vi "Laser engraver main.vi"() -> ()   [LabVIEW 2016]
uses:
  Control panel.ctl
  Data.ctl
  <vilib>/LabVIEW Interface for Arduino/Type Defs/Arduino Resource.ctl
  <vilib>/LabVIEW Interface for Arduino/Type Defs/Board Type.ctl
  States.ctl
  <vilib>/Utility/file.llb/Write Delimited Spreadsheet (string).vi
  <vilib>/LabVIEW Interface for Arduino/LabVIEW Interface for Arduino.lvlib
panel:
  in  "Szimuláció ON/OFF 4":bool
  in  "Szimuláció ON/OFF 3":bool
  in  "Szimuláció ON/OFF 2":bool
  in  "Tab Control 2":T1(tab)
  in  "Kép elhelyezése":bool
  in  "Szimuláció ON/OFF":bool
  in  "Megmunkálás":bool
  in  "Program leállítása":bool
  in  "Kezelõpult":T2={"Konverziós faktor"=1020, "Threshold"=1020, "Megjegyzések"="", "Lépés"=0, "Sebesség"=0, " X init"=0, "Y init"=0} {"Y init" min=0; "X init" min=0; "Threshold" scale=0.0..16777215.0; "Konverziós faktor" scale=1.0..100.0}
  in  "Kilépés a programból":bool
  in  "VISA resource":refnum<visa-resource-name>
  in  "Képfeldolgozás":bool
  in  "Megmunkálás leállítása":bool
  in  "Felfüggesztés/Folytatás":bool
  out "Megmunkálás kész":bool
  out "Inicializálás a kezdõpontra":bool
  out "Megmunkálás folyamatban":bool
  in  "Tab Control":T3(tab)
  out "Eredeti kép":picture
  out "Fekete-fehér tükrözött kép":picture
  out "régi x felbontás":i16
  out "régi y felbontás":i16
  out "új x felbontás / oszlopok száma":i32
  out "új y felbontás / sorok száma":i32
  out "XY Graph 2":cluster{i32[], i32[]}[](graph)
  out "XY Graph":cluster{i32, i32}[](graph)
  in  "Kép beolvasása":bool
  in  "Kezelõpult betöltése":bool
  in  "Kezelõpult mentése":bool
  in  "Szélek kijelölése":bool
  in  "Jegyzõkönyvezés":bool
  # "Lézeres gravírozás\n\nLabview-ban implementálta:\nTari Balázs"
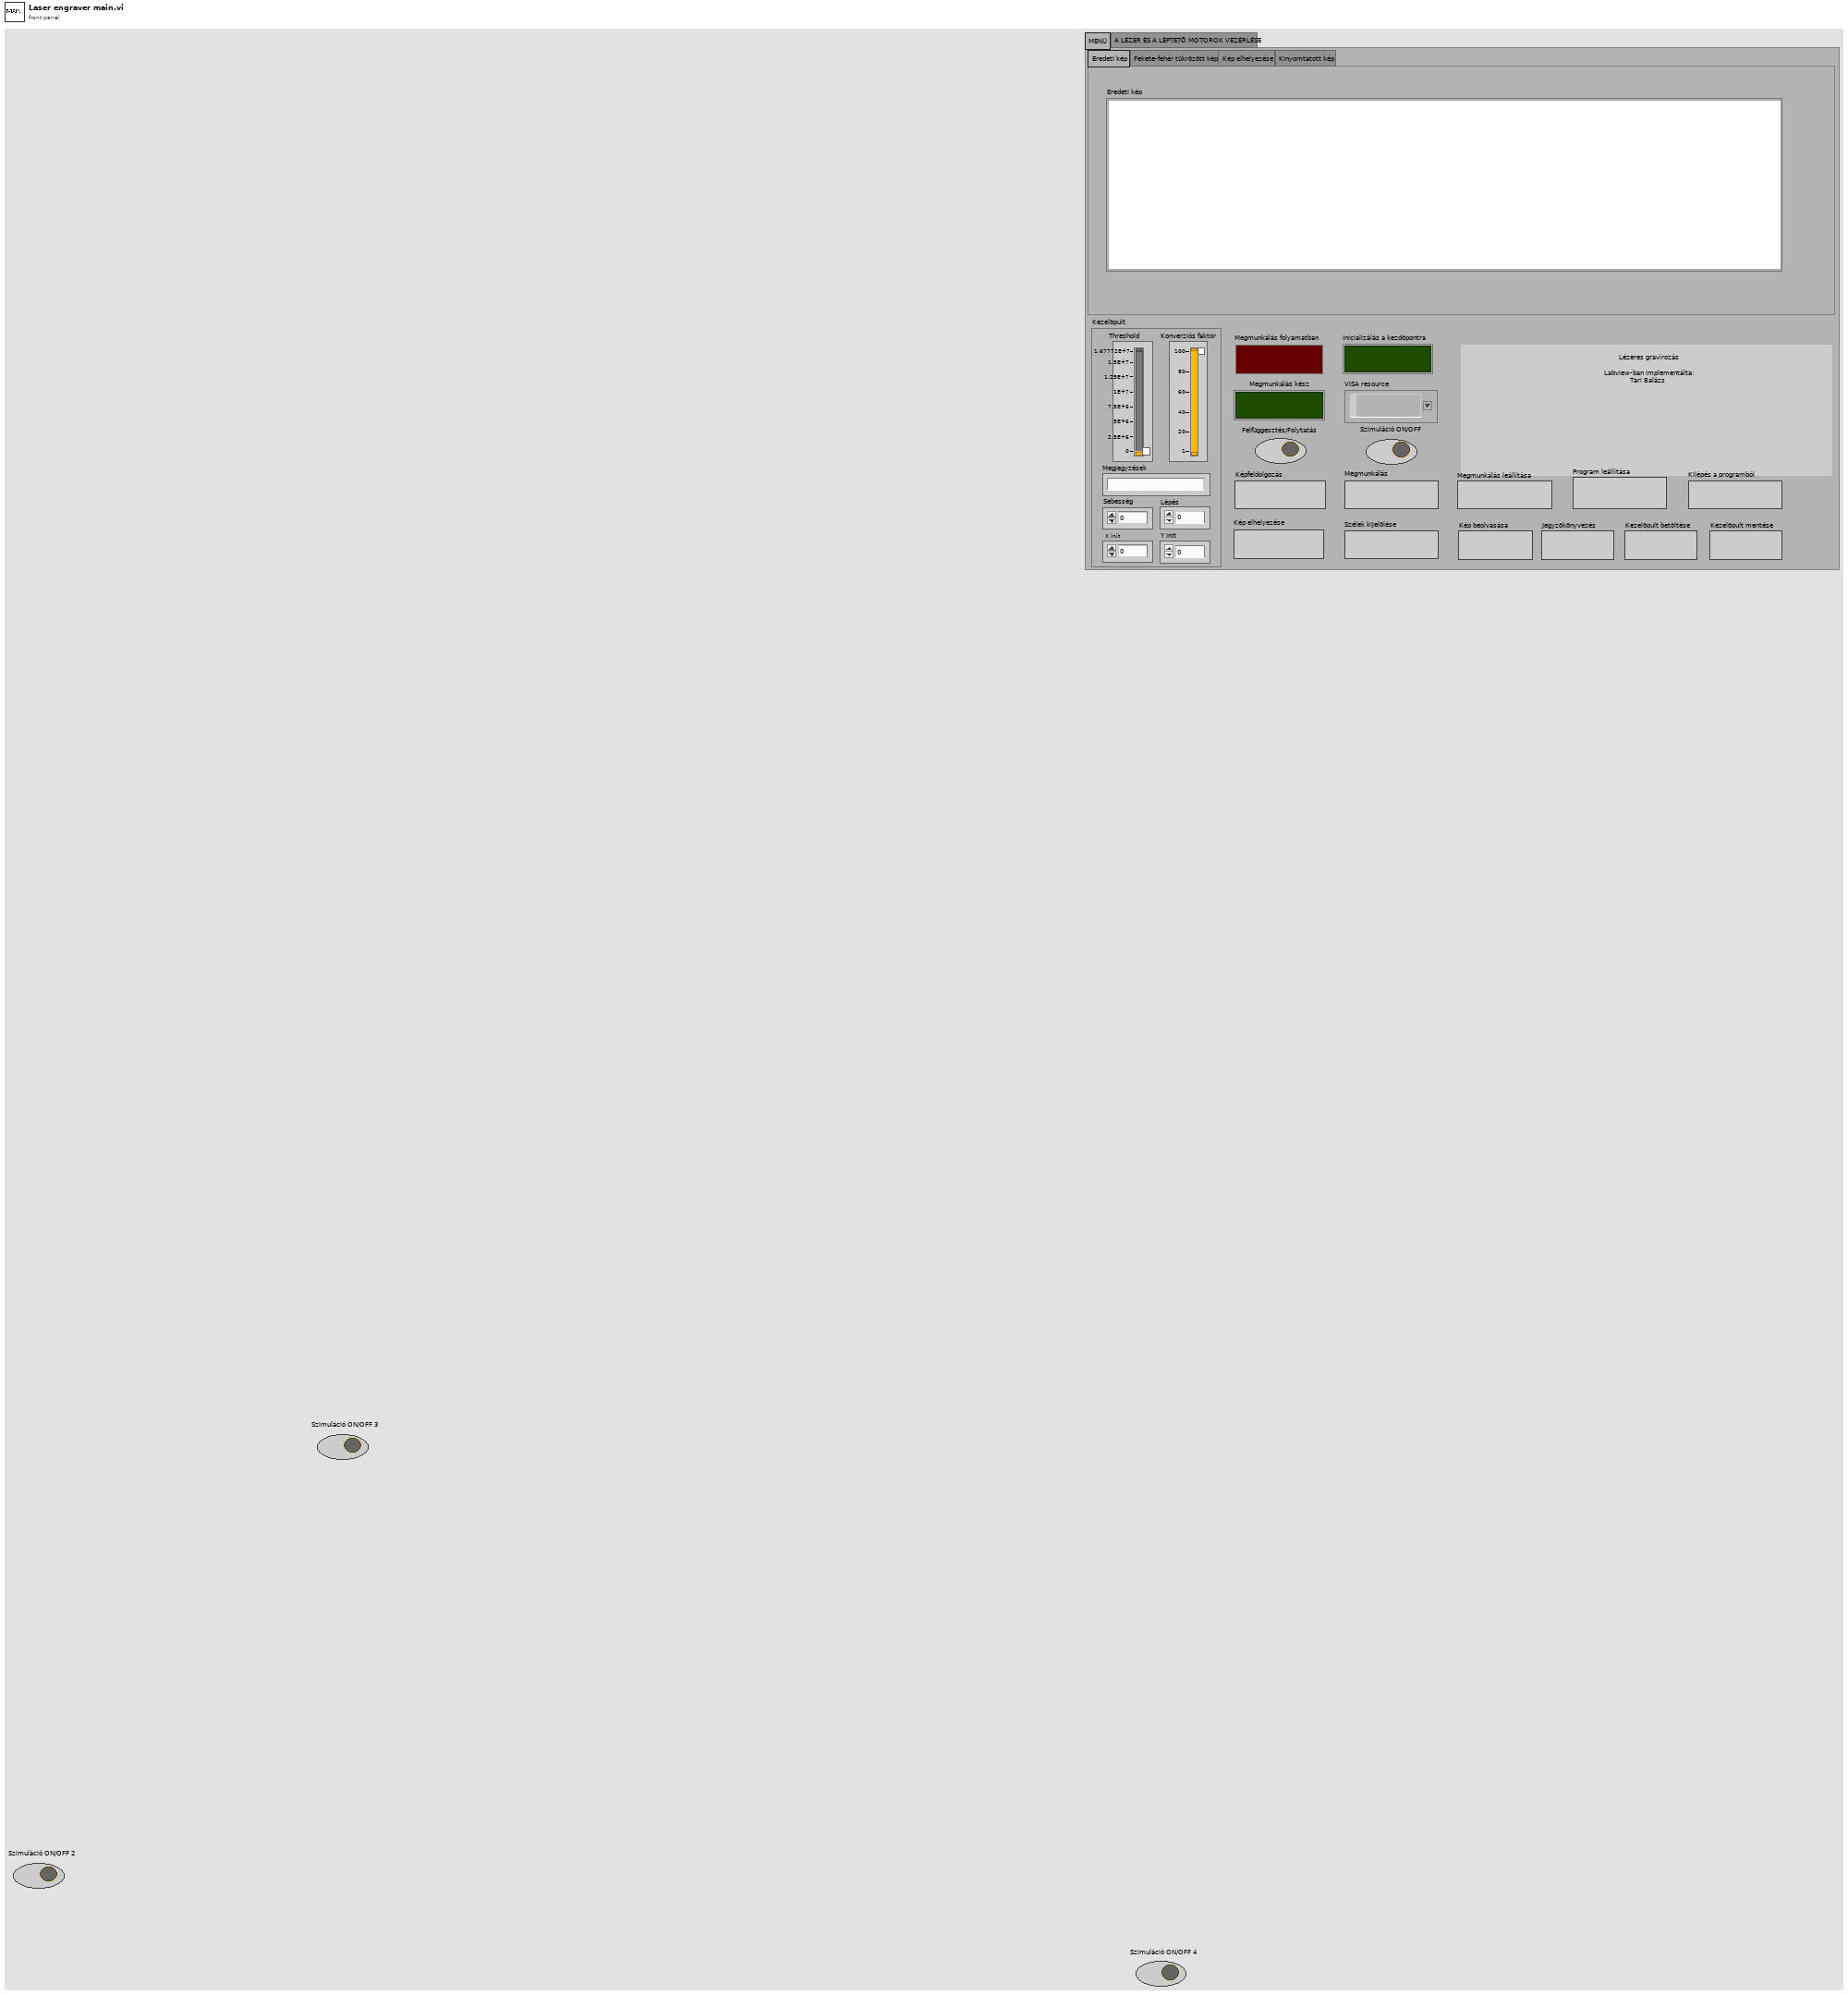
[diagram p1: front panel]
types:
  T1 = enum32{"MENÜ", "A LÉZER ÉS A LÉPTETÕ MOTOROK VEZÉRLÉSE"}
  T2 = typedef "Control panel.ctl" = cluster{"Konverziós faktor":i32, "Threshold":i32, "Megjegyzések":string, "Lépés":i32, "Sebesség":i32, " X init":i32, "Y init":i32}
  T3 = enum32{"Eredeti kép", "Fekete-fehér tükrözött kép", "Kép elhelyezése", "Kinyomtatott kép"}
  T4 = typedef "States.ctl" = enum16{"init", "init report", "init picture", "picture processing", "picture positioning", "arduino init", "mark edge", "engraving", "report", "load control panel", "save control panel", "idle", "stop"}
  T5 = typedef "Data.ctl" = cluster{"picture in":path, "config":path, "report":path, "x koordináta":i32[], "lézer vezérlés":bool[], "y koordináta":i32[], "új x felbontás / oszlopok száma":i32, "Arduino Resource":T6, "új y felbontás / sorok száma":i32, "rect":cluster{"left":i32, "top":i32, "right":i32, "bottom":i32}}
  T6 = typedef "LabVIEW Interface for Arduino.lvlib/Arduino Resource.ctl" = cluster{"VISA resource":refnum<visa-resource-name>, "Board Type":T7, "Connection Type":enum8{"USB / Serial"}, "Bytes Per Packet (15)":u8}
  T7 = typedef "LabVIEW Interface for Arduino.lvlib/Board Type.ctl" = enum16{"Uno", "Dimuelanove w/Atmega 328", "Mega 2560"}
  T8 = enum16{"open", "replace", "create", "open or create", "replace or create", "replace or create with confirmation"}
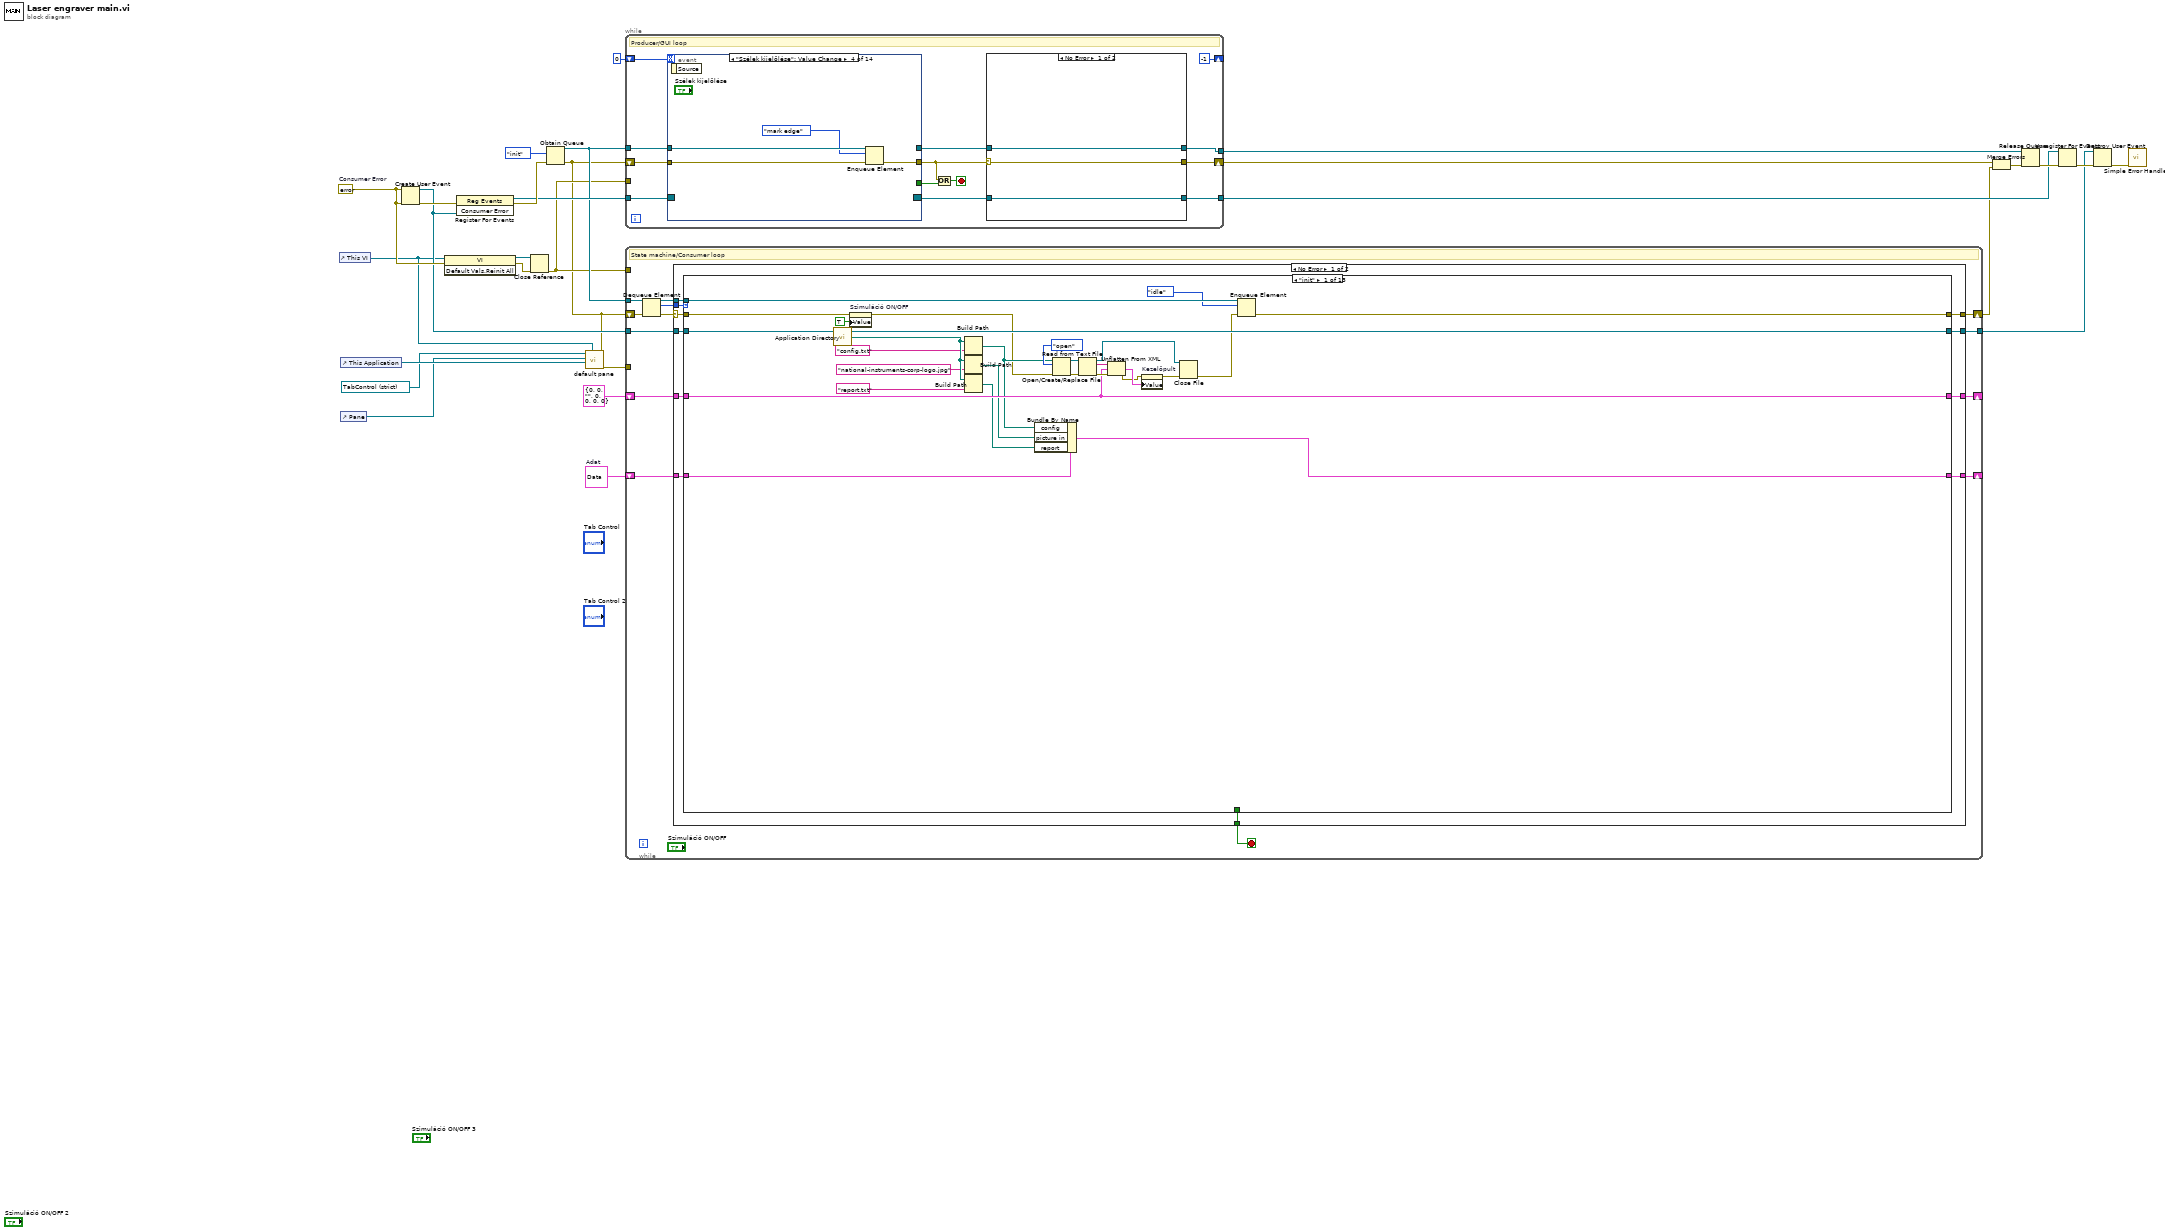
[diagram p0: block diagram]
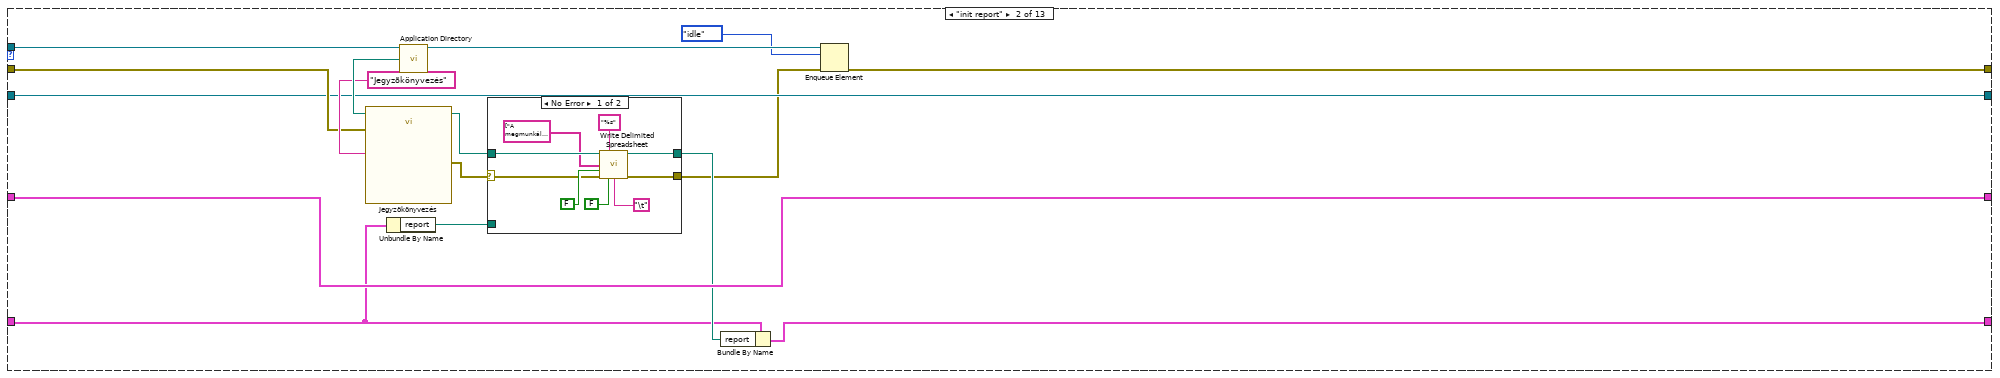
[diagram p2: hidden frame]
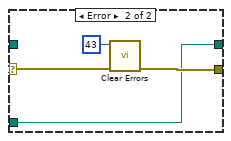
[diagram p3: hidden frame]
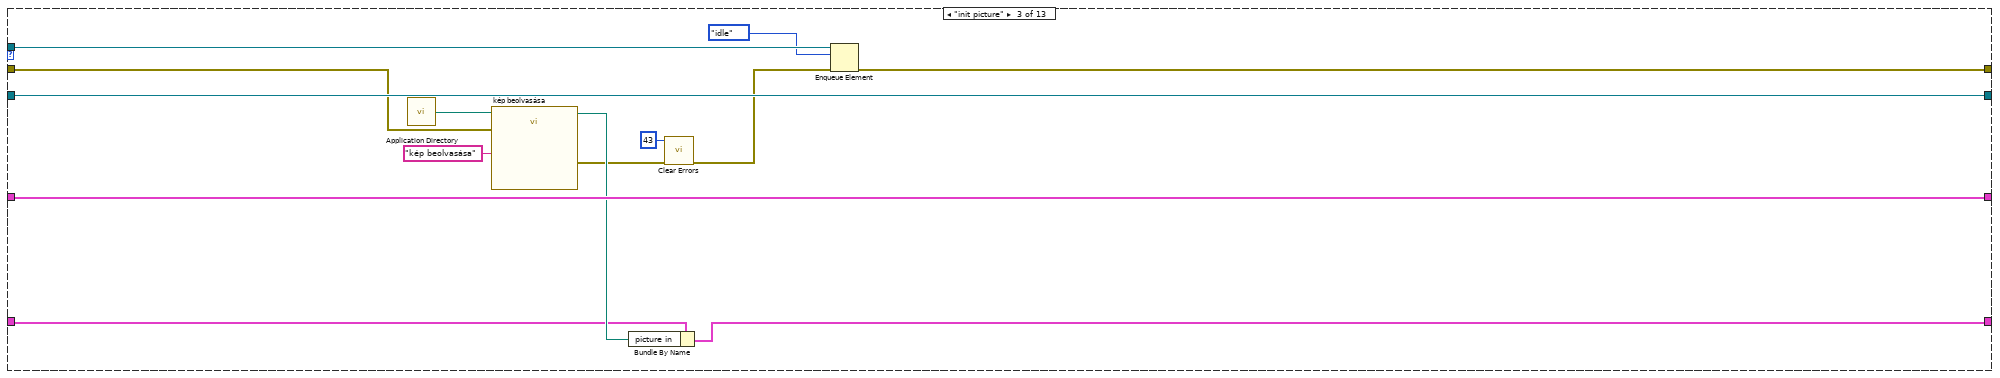
[diagram p4: hidden frame]
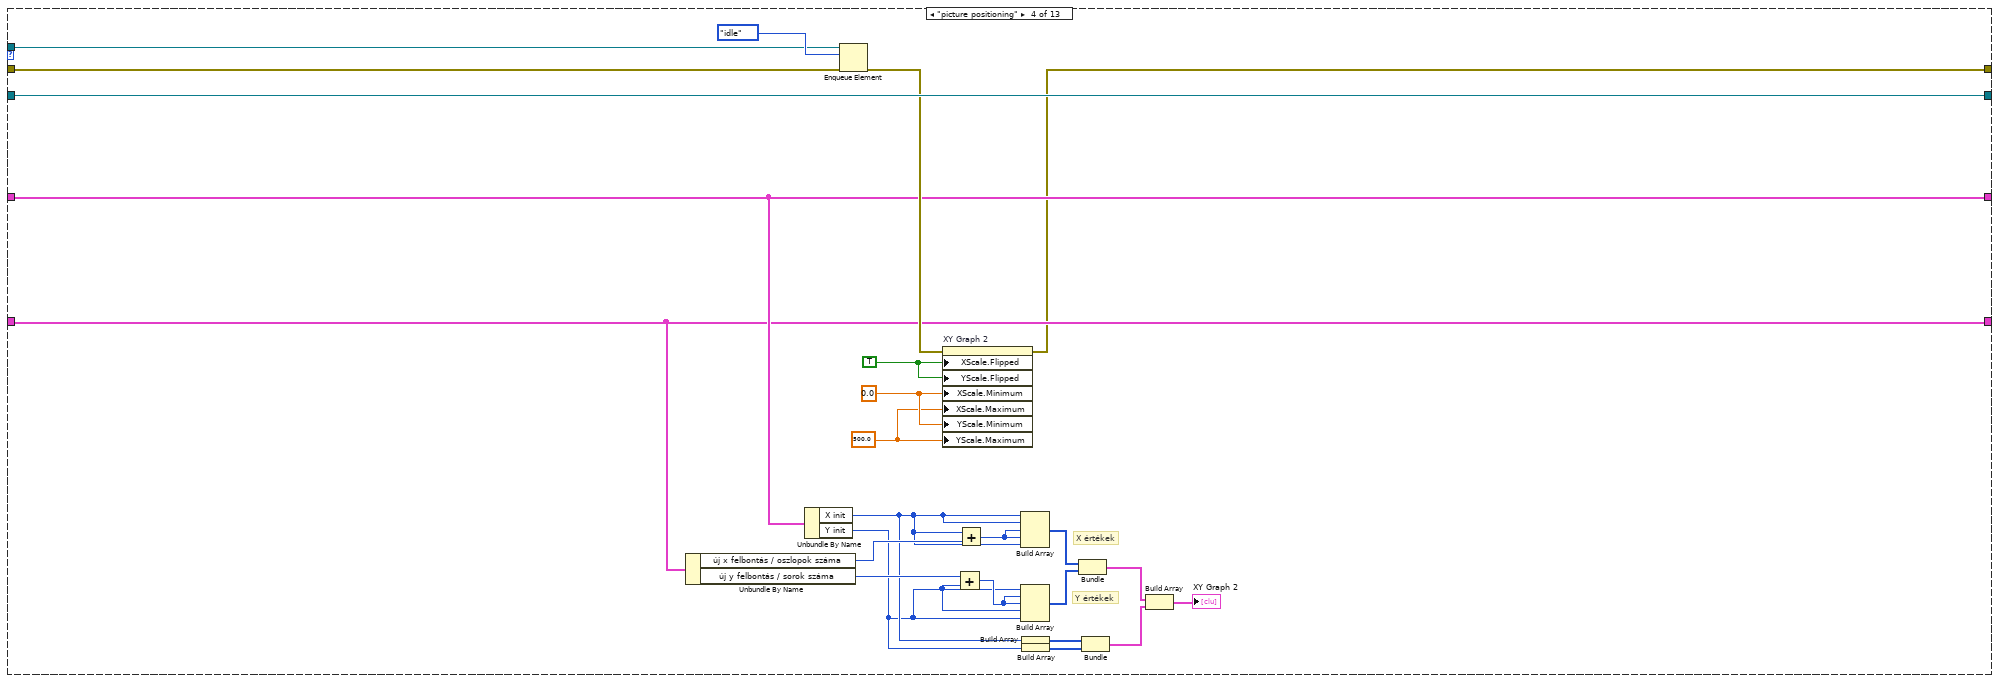
[diagram p5: hidden frame]
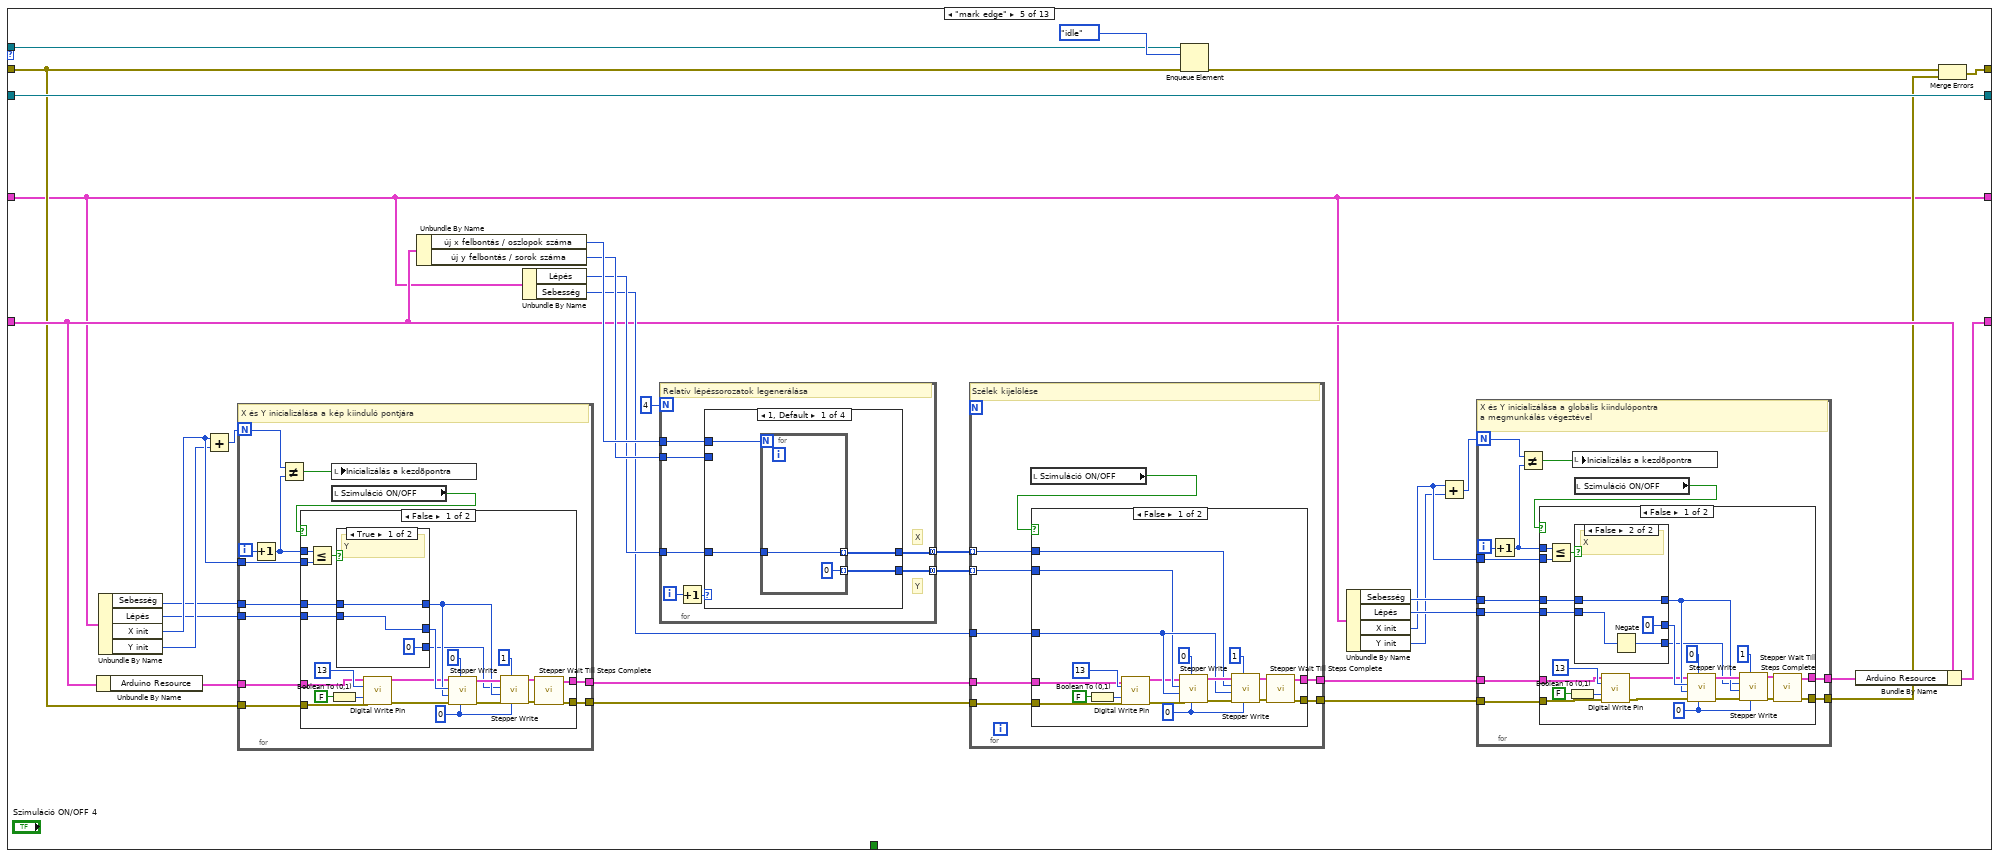
[diagram p6: hidden frame]
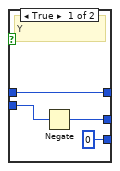
[diagram p7: hidden frame]
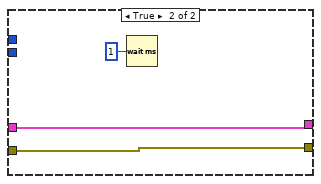
[diagram p8: hidden frame]
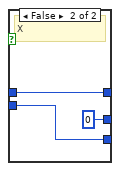
[diagram p9: hidden frame]
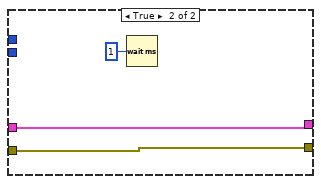
[diagram p10: hidden frame]
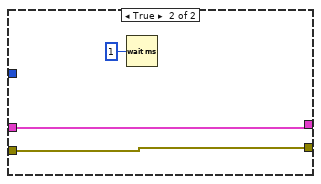
[diagram p11: hidden frame]
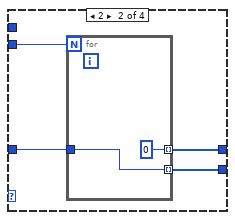
[diagram p12: hidden frame]
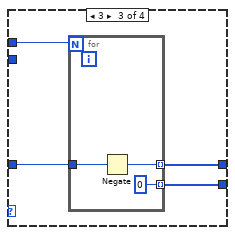
[diagram p13: hidden frame]
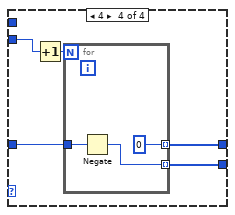
[diagram p14: hidden frame]
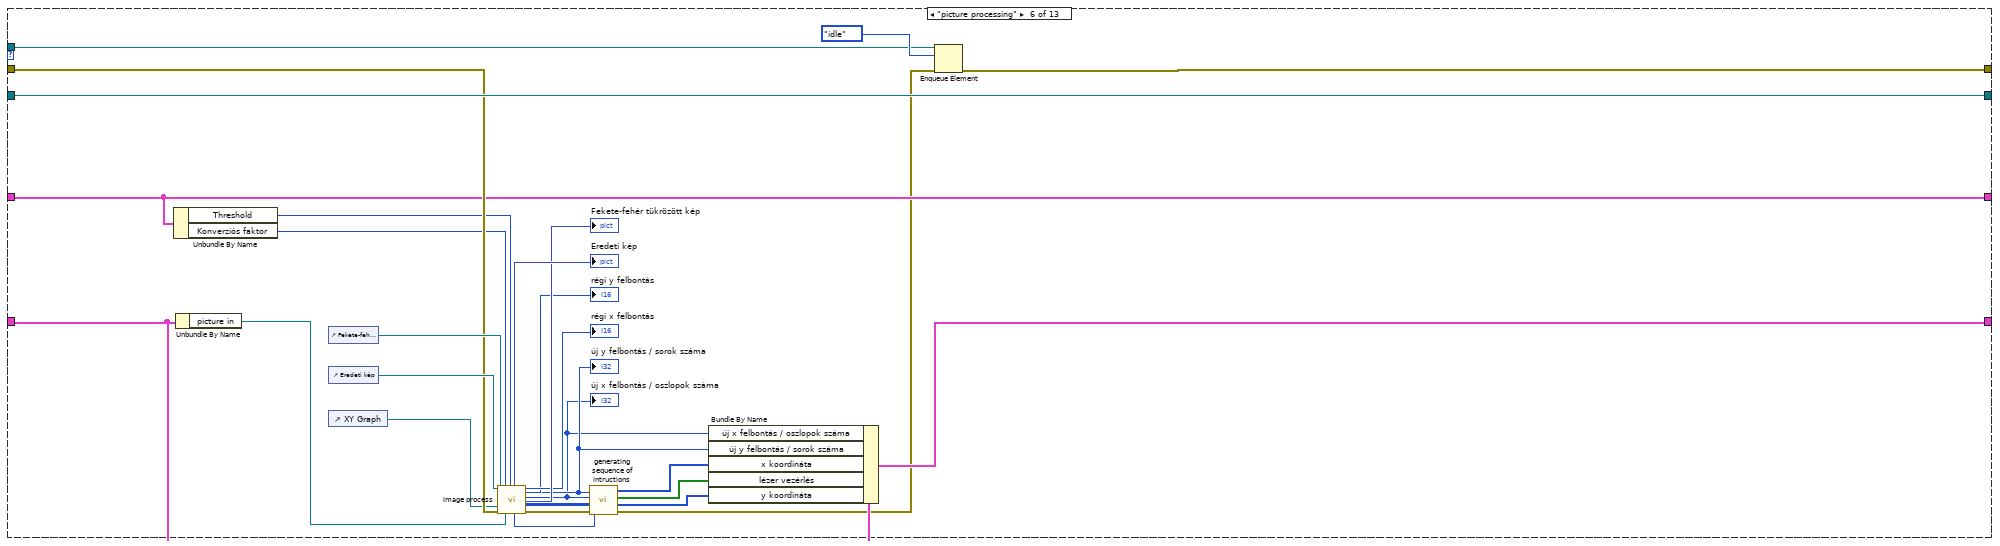
[diagram p15: hidden frame]
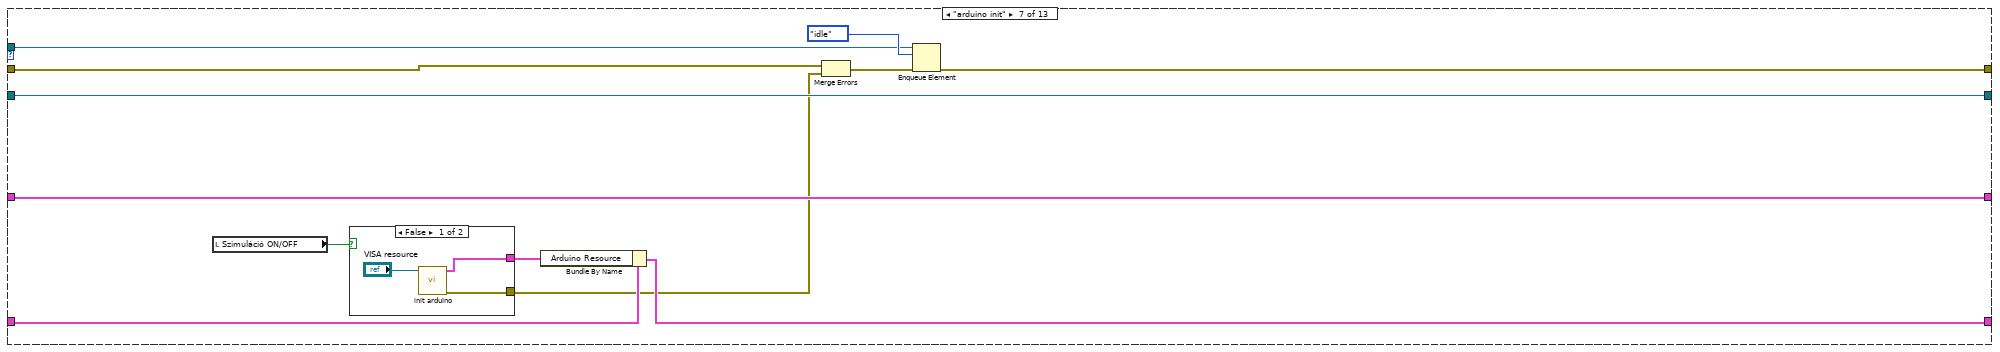
[diagram p16: hidden frame]
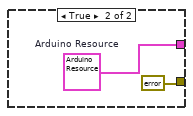
[diagram p17: hidden frame]
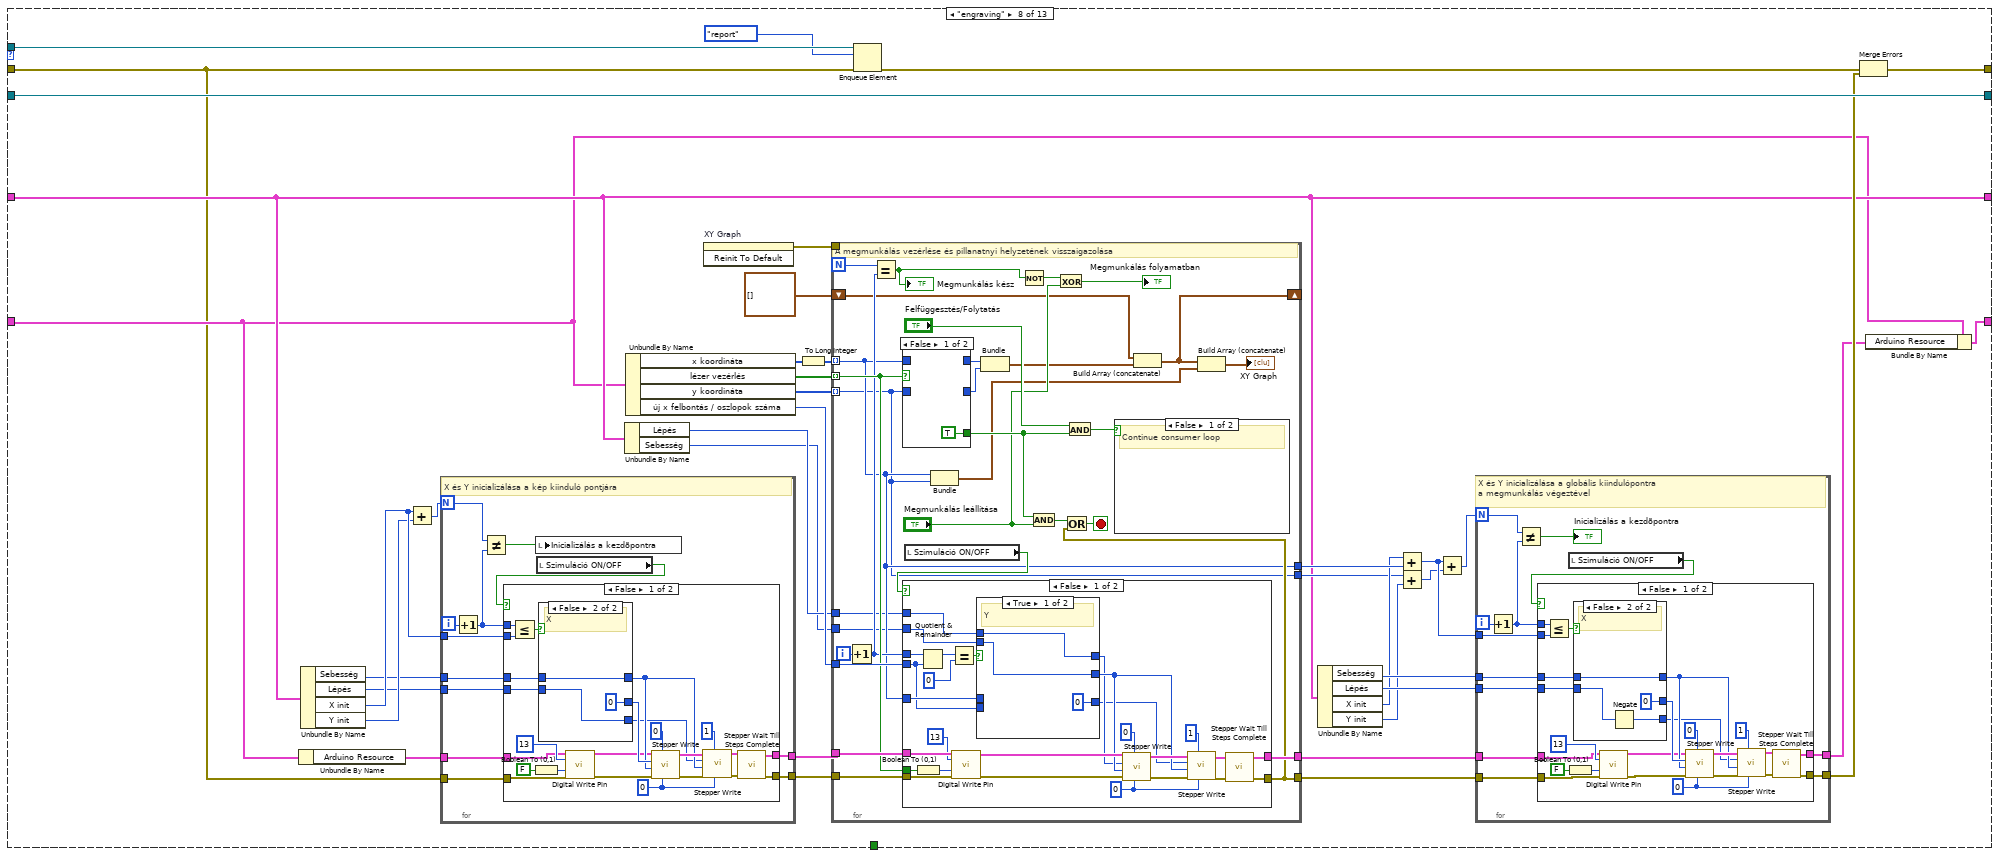
[diagram p18: hidden frame]
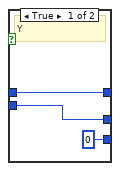
[diagram p19: hidden frame]
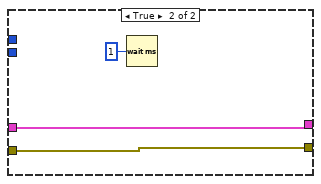
[diagram p20: hidden frame]
diagram:
  w20 = T5 {"picture in"=path "", "config"=path "", "report"=path "", "x koordináta"=[], "lézer vezérlés"=[], "y koordináta"=[], "új x felbontás / oszlopok száma"=0, "Arduino Resource"={"VISA resource"="", "Board Type"=enum."Uno", "Connection Type"=enum."USB / Serial", "Bytes Per Packet (15)"=15}, "új y felbontás / sorok száma"=0, "rect"={"left"=0, "top"=0, "right"=0, "bottom"=0}}  # Adat
  w14 = errorcluster {"status"=FALSE, "code"=0, "source"=""}  # Consumer Error
  n1 = control-ref of="This VI"() -> (w4:refnum<vi>)
  n2 = control-ref of="This Application"() -> (w5:refnum<vi>)
  n3 = control-ref of="Pane"() -> (w3:refnum<vi>)
  n4 = Create User Event(user event datatype=w14, error in=w14) -> (user event=w13:refnum<user-event>, error out=w22:errorcluster)
  n5 = invoke class="VI" method="Default Vals.Reinit All"(reference=w4, error in=w14) -> (reference out=w26:refnum<vi>, error out=w27:errorcluster)  [unwired: 1 in, 1 out]
  n6 = register-events(error in=w22, w13) -> (reference out=w21:refnum<event-registration>, error out=w28:errorcluster)  [unwired: 1 in]
  n7 = Close Reference(reference=w26, error in (no error)=w27) -> (error out=w11:errorcluster)
  n8 = Obtain Queue(element data type=States."init" ("enum"), error in (no error)=w28) -> (queue out=w12:refnum<queue>, error out=w7:errorcluster)  [unwired: 3 in, 1 out]
  n9 = call "default pane.vi"("error in (no error)"=w7, "VI Reference"=w4, "Application reference"=w5, "Pane Control"=w3, "TabControl in"=refnum<vi> refnum) -> ("error out"=w6:errorcluster)  [unwired: 6 in]
  n10 = while {
    shift-right: [w36] -> w25
    shift-left: w7 -> [w41]
    tunnel: w12 -> [w39]
    tunnel: w21 -> [w40]
    tunnel: w11 -> [_]
    tunnel: [w34] -> w19
    tunnel: [w31] -> w17
    shift-right: [-1] -> _
    shift-left: 0 -> [w30]
    stop <- w37 stop-if-true
    # "Producer/GUI loop"
    n11 = event shown="[3] \"Szélek kijelölése\": Value Change" {
      selector: w40 -> [_ _ _ _ _ _ _ _ _ _ _ _ _ _]
      dyn-events: [_ _ _ _ _ _ _ _ _ _ _ _ _ _] -> w35
      timeout: w30 -> [_ _ _ _ _ _ _ _ _ _ _ _ _ _]
      tunnel: w39 -> [w52 w58 w63 w68 w71 w78 w80 w85 w90 w95 w99 w105 w109 w138]
      tunnel: w41 -> [w53 w59 w62 w67 w72 w75 w81 w86 w91 w96 w102 w104 w110 w140]
      tunnel: [w55 w57 w61 w66 w70 w77 w83 w88 w93 w98 w101 w104 w112 w139] -> w33
      tunnel: [_ _ _ _ _ _ _ _ _ _ _ TRUE w108 _] -> w38
      tunnel: [w54 w56 _ _ w69 w76 w82 w87 w92 w97 w100 w105 w111 w137] -> w32
      event Timeout {
        n12 = event-data() -> ()  [unwired: 1 in, 1 out]
        n13 = Enqueue Element(queue=w52, element=States."init", error in (no error)=w53) -> (queue out=w54:refnum<queue>, error out=w55:errorcluster)  [unwired: 1 in, 1 out]
      }
      event "Képfeldolgozás": Value Change {
        n14 = event-data() -> ()  [unwired: 1 in, 1 out]
        n15 = Enqueue Element(queue=w58, element=States."picture processing", error in (no error)=w59) -> (queue out=w56:refnum<queue>, error out=w57:errorcluster)  [unwired: 1 in, 1 out]
      }
      event "Kép elhelyezése": Value Change {
        n16 = event-data() -> ()  [unwired: 1 in, 1 out]
        n17 = Enqueue Element(queue=w63, element=States."picture positioning", error in (no error)=w62) -> (error out=w61:errorcluster)  [unwired: 1 in, 2 out]
      }
      event "Szélek kijelölése": Value Change {
        n18 = event-data() -> ()  [unwired: 1 in, 1 out]
        n19 = Enqueue Element(queue=w68, element=States."mark edge", error in (no error)=w67) -> (error out=w66:errorcluster)  [unwired: 1 in, 2 out]
      }
      event "VISA resource", "Szimuláció ON/OFF": Value Change {
        n20 = event-data() -> ()  [unwired: 1 in, 1 out]
        n21 = Enqueue Element(queue=w71, element=States."arduino init", error in (no error)=w72) -> (queue out=w69:refnum<queue>, error out=w70:errorcluster)  [unwired: 1 in, 1 out]
      }
      event "Megmunkálás": Value Change {
        n22 = event-data() -> ()  [unwired: 1 in, 1 out]
        n23 = Enqueue Element(queue=w78, element=States."engraving", error in (no error)=w75) -> (queue out=w76:refnum<queue>, error out=w77:errorcluster)  [unwired: 1 in, 1 out]
      }
      event "Kép beolvasása": Value Change {
        n24 = event-data() -> ()  [unwired: 1 in, 1 out]
        n25 = Enqueue Element(queue=w80, element=States."init picture" ("enum"), error in (no error)=w81) -> (queue out=w82:refnum<queue>, error out=w83:errorcluster)  [unwired: 1 in, 1 out]
      }
      event "Jegyzõkönyvezés": Value Change {
        n26 = event-data() -> ()  [unwired: 1 in, 1 out]
        n27 = Enqueue Element(queue=w85, element=States."init report", error in (no error)=w86) -> (queue out=w87:refnum<queue>, error out=w88:errorcluster)  [unwired: 1 in, 1 out]
      }
      event "Kezelõpult betöltése": Value Change {
        n28 = event-data() -> ()  [unwired: 1 in, 1 out]
        n29 = Enqueue Element(queue=w90, element=States."load control panel" ("enum"), error in (no error)=w91) -> (queue out=w92:refnum<queue>, error out=w93:errorcluster)  [unwired: 1 in, 1 out]
      }
      event "Kezelõpult mentése": Value Change {
        n30 = event-data() -> ()  [unwired: 1 in, 1 out]
        n31 = Enqueue Element(queue=w95, element=States."save control panel" ("enum"), error in (no error)=w96) -> (queue out=w97:refnum<queue>, error out=w98:errorcluster)  [unwired: 1 in, 1 out]
      }
      event Value Change {
        n32 = event-data() -> ()  [unwired: 1 in, 1 out]
        n33 = Enqueue Element(queue=w99, element=States."idle" ("enum"), error in (no error)=w102) -> (queue out=w100:refnum<queue>, error out=w101:errorcluster)  [unwired: 1 in, 1 out]
      }
      event User Event {
        n34 = event-data() -> ()  [unwired: 1 in, 1 out]
      }
      event "Program leállítása": Value Change {
        n35 = event-data() -> ()  [unwired: 1 in, 1 out]
        n36 = local read "Megmunkálás folyamatban"() -> (w107:bool)
        n37 = case shown="False" w107 {
          tunnel: [w118 w135] -> w112
          tunnel: [w117 w134] -> w111
          tunnel: w110 -> [w116 w135]
          tunnel: w109 -> [w115 w134]
          tunnel: [w114 _] -> w108
          frame False {
            n38 = Two Button Dialog(message="Biztosan leállítja a programot?", 1:"Mégse" ("F button name (\"Cancel\")"), 2:"Igen" ("T button name (\"OK\")")) -> (T button?=w122:bool)
            n39 = case shown="True" w122 {
              tunnel: [w126 w131] -> w123
              tunnel: w116 -> [w126 w131]
              tunnel: [w125 w130] -> w124
              tunnel: w115 -> [w125 w130]
              tunnel: [States."idle" ("enum") States."stop" ("enum")] -> w113
              tunnel: [_ TRUE] -> w114
              frame False {
              }
              frame True {
              }
            }
            n40 = Enqueue Element(queue=w124, element=w113, error in (no error)=w123) -> (queue out=w117:refnum<queue>, error out=w118:errorcluster)  [unwired: 1 in, 1 out]
          }
          frame True {
            n41 = One Button Dialog(message="Megmunkálás folyamatban!\nA program leállításához elõbb \nállítsa le a megmunkálást!", button name ("OK")="OK") -> ()  [unwired: 1 out]
          }
        }
      }
      event "Kilépés a programból": Value Change {
        n42 = event-data() -> ()  [unwired: 1 in, 1 out]
        n43 = local read "Megmunkálás folyamatban"() -> (w136:bool)
        n44 = case shown="True" w136 {
          tunnel: w140 -> [w148 w158]
          tunnel: [w147 w158] -> w139
          tunnel: w138 -> [w146 w159]
          tunnel: [w145 w159] -> w137
          frame False {
            n45 = Two Button Dialog(message="Biztosan kilép a programból?", 1:"Mégse" ("F button name (\"Cancel\")"), 2:"Kilépés" ("T button name (\"OK\")")) -> (T button?=w141:bool)
            n46 = case shown="True" w141 {
              tunnel: w148 -> [w153 w155]
              tunnel: [w152 w155] -> w147
              tunnel: w146 -> [w151 w154]
              tunnel: [w150 w154] -> w145
              frame False {
                n47 = Enqueue Element(queue=w151, element=States."idle" ("enum"), error in (no error)=w153) -> (queue out=w150:refnum<queue>, error out=w152:errorcluster)  [unwired: 1 in, 1 out]
              }
              frame True {
                n48 = Quit LabVIEW() -> ()  [unwired: 1 in]
              }
            }
          }
          frame True {
            n49 = One Button Dialog(message="Megmunkálás folyamatban!\nA programból való kilépéshez \nelõbb állítsa le a megmunkálást!", button name ("OK")="OK") -> ()  [unwired: 1 out]
          }
        }
      }
    }
    n50 = Or(x=w33, y=w38) -> (x .or. y?=w37:bool)
    n51 = case shown="No Error" w33 {
      selector: w33 -> [w44 w46]
      tunnel: [w44 w45] -> w36
      tunnel: w32 -> [w43 w50]
      tunnel: [w43 w49] -> w31
      tunnel: [w42 w48] -> w34
      tunnel: w35 -> [w42 w48]
      frame No Error {
      }
      frame Error {
        n52 = Enqueue Element At Opposite End(queue=w50, element=States."stop" ("enum"), error in (no error)=w46) -> (queue out=w49:refnum<queue>, error out=w45:errorcluster)  [unwired: 1 in, 1 out]
      }
    }
  }
  n53 = while {
    tunnel: w12 -> [w172]
    tunnel: w13 -> [w168]
    shift-right: [w169] -> w15
    shift-left: w7 -> [w171]
    tunnel: [w167] -> w9
    tunnel: w11 -> [_]
    shift-right: [w163] -> _
    shift-left: T2 {"Konverziós faktor"=0, "Threshold"=0, "Megjegyzések"="", "Lépés"=0, "Sebesség"=0, " X init"=0, "Y init"=0} ("Kezelõpult") -> [w164]
    shift-right: [w161] -> _
    shift-left: w20 -> [w162]
    tunnel: w6 -> [_]
    stop <- w170 stop-if-true
    # "State machine/Consumer loop"
    n54 = Dequeue Element(queue=w172, error in (no error)=w171) -> (queue out=w165:refnum<queue>, element=w160:T4, error out=w166:errorcluster)  [unwired: 1 in, 1 out]
    n55 = case shown="No Error" w166 {
      selector: w166 -> [w173 w818]
      tunnel: w160 -> [w183 _]
      tunnel: [w182 TRUE] -> w170
      tunnel: [w181 w820] -> w169
      tunnel: w168 -> [w180 w824]
      tunnel: [w179 w823] -> w167
      tunnel: w165 -> [w178 _]
      tunnel: w164 -> [w177 w821]
      tunnel: [w176 w821] -> w163
      tunnel: w162 -> [w175 w817]
      tunnel: [w174 w817] -> w161
      frame No Error {
        n56 = case shown="\"init\"" w183 {
          tunnel: w173 -> [w185 w221 w247 w274 w288 w484 w498 w510 w722 w742 w775 w799 w804]
          tunnel: [w209 w223 w252 w262 w287 w470 w494 w540 w734 w750 w783 w799 w806] -> w181
          tunnel: [_ _ _ _ _ _ _ _ _ _ _ _ TRUE] -> w182
          tunnel: w180 -> [w210 w220 w250 w276 w309 w492 w502 w548 w735 w748 w782 w802 w809]
          tunnel: [w210 w220 w250 w276 w309 w492 w502 w548 w735 w748 w782 w802 w809] -> w179
          tunnel: w178 -> [w208 w222 w243 w273 w304 w468 w493 w547 w733 w749 w779 _ _]
          tunnel: w177 -> [w199 w218 w251 w268 w277 w475 w503 w512 w725 w747 w780 _ w808]
          tunnel: [w199 w218 w251 w268 w277 w475 w503 w512 w725 w747 w780 "Kezelõpult" w808] -> w176
          tunnel: w175 -> [w207 w212 w245 w267 w291 w478 w500 w511 w732 w738 w770 w800 w807]
          tunnel: [w206 w219 w244 w267 w300 w480 w499 w538 w732 w741 w772 w800 w807] -> w174
          frame "init" {
            n57 = call <vilib>:"Application Directory.vi"() -> ("Application Directory"=w198:path)
            n58 = property on="Szimuláció ON/OFF" class="Bool (strict)"(error in=w185, "Value"=TRUE ("Szimuláció ON/OFF")) -> (error out=w184:errorcluster)  [unwired: 1 in, 1 out]
            n59 = Build Path(base path=w198, name or relative path="config.txt") -> (appended path=w192:path)
            n60 = Build Path(base path=w198, name or relative path="national-instruments-corp-logo.jpg") -> (appended path=w194:path)
            n61 = Build Path(base path=w198, name or relative path="report.txt") -> (appended path=w193:path)
            n62 = Bundle By Name(cluster=w207, "config"=w192, "picture in"=w194, "report"=w193) -> (w206:T5)
            n63 = Open/Create/Replace File(file path (use dialog)=w192, error in=w184, operation (0:open)=T8."open") -> (refnum out=w202:refnum<file>, error out=w203:errorcluster)  [unwired: 3 in, 1 out]
            n64 = Read from Text File(file (use dialog)=w202, error in=w203) -> (refnum out=w200:refnum<file>, text=w204:string, error out=w205:errorcluster)  [unwired: 2 in, 1 out]
            n65 = Unflatten From XML(xml string=w204, type=w199, error in (no error)=w205) -> (value=w191:T2, error out=w190:errorcluster)
            n66 = property on="Kezelõpult" class="Clust (strict)"(error in=w190, "Value"=w191) -> (error out=w189:errorcluster)  [unwired: 1 in, 1 out]
            n67 = Close File(refnum=w200, error in=w189) -> (error out=w187:errorcluster)  [unwired: 1 out]
            n68 = Enqueue Element(queue=w208, element=States."idle" ("enum"), error in (no error)=w187) -> (error out=w209:errorcluster)  [unwired: 1 in, 2 out]
          }
          frame "init report" {
            n69 = Unbundle By Name(w212) -> ("report"=w211:path)
            n70 = call <vilib>:"Application Directory.vi"() -> ("Application Directory"=w225:path)
            n71 = call "Jegyzõkönyvezés"("start path"=w225, "button label"="Jegyzõkönyvezés", "error in"=w221) -> ("selected path"=w217:path, "error out"=w213:errorcluster)  [unwired: 9 in, 2 out]
            n72 = case shown="No Error" w213 {
              selector: w213 -> [w230 w238]
              tunnel: w217 -> [w229 _]
              tunnel: [w227 w235] -> w216
              tunnel: [w228 w236] -> w214
              tunnel: w211 -> [_ w235]
              frame No Error {
                n73 = call-poly <vilib>:"Write Delimited Spreadsheet.vi"("file path (dialog if empty)"=w229, "format (%s)"="%s", "1D data"=string[] ["A megmunkálás idõpontja ", "Konfigurációs fájl", "Megjegyzések"], "append to file? (new file:F)"=FALSE, "error in (no error)"=w230, "transpose? (no:F)"=FALSE ("append to file? (new file:F)"), "delimiter (\\t)"="\t") -> ("new file path (Not A Path if cancelled)"=w227:path, "error out"=w228:errorcluster)  [unwired: 7 in]
              }
              frame Error {
                n74 = call <vilib>:"Clear Errors.vi"("error in (no error)"=w238, "specific error code to clear (0: all)"=43) -> ("error out"=w236:errorcluster)  [unwired: 4 in, 1 out]
              }
            }
            n75 = Bundle By Name(cluster=w212, "report"=w216) -> (w219:T5)
            n76 = Enqueue Element(queue=w222, element=States."idle" ("enum"), error in (no error)=w214) -> (error out=w223:errorcluster)  [unwired: 1 in, 2 out]
          }
          frame "init picture" {
            n77 = call <vilib>:"Application Directory.vi"() -> ("Application Directory"=w249:path)
            n78 = call "kép beolvasása"("start path"=w249, "button label"="kép beolvasása", "error in"=w247) -> ("selected path"=w246:path, "error out"=w240:errorcluster)  [unwired: 9 in, 2 out]
            n79 = Bundle By Name(cluster=w245, "picture in"=w246) -> (w244:T5)
            n80 = call <vilib>:"Clear Errors.vi"("error in (no error)"=w240, "specific error code to clear (0: all)"=43) -> ("error out"=w239:errorcluster)  [unwired: 4 in, 1 out]
            n81 = Enqueue Element(queue=w243, element=States."idle" ("enum"), error in (no error)=w239) -> (error out=w252:errorcluster)  [unwired: 1 in, 2 out]
          }
          frame "picture positioning" {
            w270 = 500.0 ("X Scale.Range:Minimum")
            w271 = 0.0 ("X Scale.Range:Minimum")
            w272 = TRUE ("X Scale.Flipped")
            # "Y értékek"
            # "X értékek"
            n82 = Unbundle By Name(w267) -> ("új x felbontás / oszlopok száma"=w263:i32, "új y felbontás / sorok száma"=w264:i32)
            n83 = Unbundle By Name(w268) -> ("X init"=w254:i32, "Y init"=w253:i32)
            n84 = Enqueue Element(queue=w273, element=States."idle" ("enum"), error in (no error)=w274) -> (error out=w269:errorcluster)  [unwired: 1 in, 2 out]
            n85 = property on="XY Graph 2" class="XYGraph (strict)"(error in=w269, "XScale.Flipped"=w272, "YScale.Flipped"=w272, "XScale.Minimum"=w271, "XScale.Maximum"=w270, "YScale.Minimum"=w271, "YScale.Maximum"=w270) -> (error out=w262:errorcluster)  [unwired: 1 in, 1 out]
            n86 = Add(x=w264, y=w253) -> (x+y=w260:i32)
            n87 = Add(x=w254, y=w263) -> (x+y=w261:i32)
            n88 = Build Array(w254, w254, w261, w261, w254) -> (w265:i32[])
            n89 = Build Array(w253, w260, w260, w253, w253) -> (w266:i32[])
            n90 = Build Array(w254) -> (w259:i32[])
            n91 = Build Array(w253) -> (w258:i32[])
            n92 = Bundle(w265, w266) -> (w256:cluster{i32[], i32[]})  [unwired: 1 in]
            n93 = Bundle(w259, w258) -> (w257:cluster{i32[], i32[]})  [unwired: 1 in]
            n94 = Build Array(w256, w257) -> (→"XY Graph 2":cluster{i32[], i32[]}[])
          }
          frame "mark edge" {
            n95 = Unbundle By Name(w291) -> ("Arduino Resource"=w297:T6)
            n96 = Unbundle By Name(w277) -> ("Sebesség"=w293:i32, "Lépés"=w294:i32, "X init"=w296:i32, "Y init"=w295:i32)
            n97 = Add(x=w296, y=w295) -> (x+y=w292:i32)
            n98 = for {
              N: w292 -> [w362]
              tunnel: w296 -> [w368]
              tunnel: [w365] -> w290
              tunnel: [w364] -> w289
              tunnel: w288 -> [w367]
              tunnel: w297 -> [w366]
              tunnel: w293 -> [w360]
              tunnel: w294 -> [w359]
              i -> [w363]
              # "X és Y inicializálása a kép kiinduló pontjára"
              n99 = Increment(x=w363) -> (x+1=w361:i32)
              n100 = Not Equal?(x=w362, y=w361) -> (x != y?=w357:bool)
              n101 = local write "Inicializálás a kezdõpontra"(w357) -> ()
              n102 = local read "Szimuláció ON/OFF"() -> (w358:bool)
              n103 = case shown="False" w358 {
                tunnel: w368 -> [w392 _]
                tunnel: w367 -> [w372 w401]
                tunnel: w366 -> [w369 w400]
                tunnel: [w389 w400] -> w365
                tunnel: [w388 w401] -> w364
                tunnel: w361 -> [w387 _]
                tunnel: w360 -> [w377 _]
                tunnel: w359 -> [w376 _]
                frame False {
                  w379 = i16 0 ("Set Acceleration (0 to disable)")
                  n104 = Less Or Equal?(x=w387, y=w392) -> (x <= y?=w391:bool)
                  n105 = Boolean To (0,1)(Boolean=FALSE) -> (0, 1=w375:i16)
                  n106 = case shown="True" w391 {
                    tunnel: [w395 w398] -> w380
                    tunnel: [w393 0] -> w390
                    tunnel: [0 w396] -> w378
                    tunnel: w377 -> [w395 w398]
                    tunnel: w376 -> [w393 w396]
                    frame True {
                      # "Y"
                    }
                    frame False {
                      # "X"
                    }
                  }
                  n107 = call <vilib>:"Digital Write Pin.vi"("Arduino Resource"=w369, "Digital I/O Pin (0)"=u8 13, "Value (0)"=w375, "error in"=w372) -> ("Arduino Resource"=w371:T6, "error out"=w370:errorcluster)  [unwired: 10 in]
                  n108 = call <vilib>:"Stepper Write.vi"("Set Acceleration (0 to disable)"=w379, "Stepper #"=u8 0, "error in"=w370, "Set Speed (Steps per Second)"=w380, "# of Steps to Move"=w390, "Arduino Resource"=w371) -> ("error out"=w386:errorcluster, "Arduino Resource Out"=w385:T6)  [unwired: 4 in]
                  n109 = call <vilib>:"Stepper Write.vi"("Set Acceleration (0 to disable)"=w379, "Stepper #"=u8 1, "error in"=w386, "Set Speed (Steps per Second)"=w380, "# of Steps to Move"=w378, "Arduino Resource"=w385) -> ("error out"=w383:errorcluster, "Arduino Resource Out"=w384:T6)  [unwired: 4 in]
                  n110 = call <vilib>:"Stepper Wait Till Steps Complete.vi"("error in"=w383, "Arduino Resource In"=w384) -> ("error out"=w388:errorcluster, "Arduino Resource Out"=w389:T6)  [unwired: 8 in]
                }
                frame True {
                  n111 = Wait (ms)(milliseconds to wait=u32 1) -> ()  [unwired: 1 out]
                }
              }
            }
            n112 = Unbundle By Name(w291) -> ("új x felbontás / oszlopok száma"=w307:i32, "új y felbontás / sorok száma"=w306:i32)
            n113 = Unbundle By Name(w277) -> ("Lépés"=w302:i32, "Sebesség"=w301:i32)
            n114 = for {
              N: 4 -> [_]
              tunnel: w307 -> [w436]
              tunnel: w306 -> [w435]
              tunnel: w302 -> [w434]
              tunnel: [w433] -> w299 mode=concatenating
              tunnel: [w432] -> w298 mode=concatenating
              i -> [w438]
              # "X"
              # "Y"
              # "Relatív lépéssorozatok legenerálása"
              n115 = Increment(x=w438) -> (x+1=w437:i32)
              n116 = case shown="1, Default" w437 {
                tunnel: w436 -> [w442 _ w454 _]
                tunnel: w435 -> [_ w448 _ w462]
                tunnel: w434 -> [w441 w447 w453 w460]
                tunnel: [w440 w446 w452 w459] -> w433
                tunnel: [w439 w445 w451 w458] -> w432
                frame 1, Default {
                  n117 = for {
                    N: w442 -> [_]
                    tunnel: w441 -> [w444]
                    tunnel: [w444] -> w440 mode=indexing
                    tunnel: [0 ("Lépés")] -> w439 mode=indexing
                    # "Y koordináták generálása\nsorok"
                  }
                }
                frame 2 {
                  n118 = for {
                    N: w448 -> [_]
                    tunnel: w447 -> [w450]
                    tunnel: [0 ("Lépés")] -> w446 mode=indexing
                    tunnel: [w450] -> w445 mode=indexing
                    # "Y koordináták generálása\nsorok"
                  }
                }
                frame 3 {
                  n119 = for {
                    N: w454 -> [_]
                    tunnel: w453 -> [w457]
                    tunnel: [w456] -> w452 mode=indexing
                    tunnel: [0 ("-x")] -> w451 mode=indexing
                    # "Y koordináták generálása\nsorok"
                    n120 = Negate(x=w457) -> (-x=w456:i32)
                  }
                }
                frame 4 {
                  n121 = Increment(x=w462) -> (x+1=w461:i32)
                  n122 = for {
                    N: w461 -> [_]
                    tunnel: w460 -> [w465]
                    tunnel: [0 ("Lépés")] -> w459 mode=indexing
                    tunnel: [w463] -> w458 mode=indexing
                    # "Y koordináták generálása\nsorok"
                    n123 = Negate(x=w465) -> (-x=w463:i32)
                  }
                }
              }
            }
            n124 = for {
              tunnel: [w407] -> w283
              tunnel: [w406] -> w282
              tunnel: w289 -> [w409]
              tunnel: w290 -> [w408]
              tunnel: w301 -> [w405]
              tunnel: w299 -> [w404] mode=indexing
              tunnel: w298 -> [w403] mode=indexing
              # "Szélek kijelölése"
              n125 = local read "Szimuláció ON/OFF"() -> (w402:bool)
              n126 = case shown="False" w402 {
                tunnel: w409 -> [w413 w431]
                tunnel: w408 -> [w412 w430]
                tunnel: [w428 w430] -> w407
                tunnel: [w427 w431] -> w406
                tunnel: w405 -> [w419 _]
                tunnel: w404 -> [w418 _]
                tunnel: w403 -> [w417 _]
                frame False {
                  w420 = i16 0 ("Set Acceleration (0 to disable)")
                  n127 = Boolean To (0,1)(Boolean=FALSE) -> (0, 1=w416:i16)
                  n128 = call <vilib>:"Digital Write Pin.vi"("Arduino Resource"=w412, "Digital I/O Pin (0)"=u8 13, "Value (0)"=w416, "error in"=w413) -> ("Arduino Resource"=w411:T6, "error out"=w410:errorcluster)  [unwired: 10 in]
                  n129 = call <vilib>:"Stepper Write.vi"("Set Acceleration (0 to disable)"=w420, "Stepper #"=u8 0, "error in"=w410, "Set Speed (Steps per Second)"=w419, "# of Steps to Move"=w417, "Arduino Resource"=w411) -> ("error out"=w426:errorcluster, "Arduino Resource Out"=w425:T6)  [unwired: 4 in]
                  n130 = call <vilib>:"Stepper Write.vi"("Set Acceleration (0 to disable)"=w420, "Stepper #"=u8 1, "error in"=w426, "Set Speed (Steps per Second)"=w419, "# of Steps to Move"=w418, "Arduino Resource"=w425) -> ("error out"=w423:errorcluster, "Arduino Resource Out"=w424:T6)  [unwired: 4 in]
                  n131 = call <vilib>:"Stepper Wait Till Steps Complete.vi"("error in"=w423, "Arduino Resource In"=w424) -> ("error out"=w427:errorcluster, "Arduino Resource Out"=w428:T6)  [unwired: 8 in]
                }
                frame True {
                  n132 = Wait (ms)(milliseconds to wait=u32 1) -> ()  [unwired: 1 out]
                }
              }
            }
            n133 = Enqueue Element(queue=w304, element=States."idle" ("enum"), error in (no error)=w288) -> (error out=w303:errorcluster)  [unwired: 1 in, 2 out]
            n134 = Unbundle By Name(w277) -> ("Sebesség"=w285:i32, "Lépés"=w286:i32, "X init"=w279:i32, "Y init"=w278:i32)
            n135 = Add(x=w279, y=w278) -> (x+y=w284:i32)
            n136 = for {
              N: w284 -> [w315]
              tunnel: w279 -> [w321]
              tunnel: [w318] -> w281
              tunnel: [w317] -> w280
              tunnel: w282 -> [w320]
              tunnel: w283 -> [w319]
              tunnel: w285 -> [w313]
              tunnel: w286 -> [w312]
              i -> [w316]
              # "X és Y inicializálása a globális kiindulópontra\na megmunkálás végeztével"
              n137 = Increment(x=w316) -> (x+1=w314:i32)
              n138 = Not Equal?(x=w315, y=w314) -> (x != y?=w310:bool)
              n139 = local write "Inicializálás a kezdõpontra"(w310) -> ()
              n140 = local read "Szimuláció ON/OFF"() -> (w311:bool)
              n141 = case shown="False" w311 {
                tunnel: w321 -> [w345 _]
                tunnel: w320 -> [w326 w356]
                tunnel: w319 -> [w323 w355]
                tunnel: [w342 w355] -> w318
                tunnel: [w341 w356] -> w317
                tunnel: w314 -> [w340 _]
                tunnel: w313 -> [w330 _]
                tunnel: w312 -> [w329 _]
                frame False {
                  w332 = i16 0 ("Set Acceleration (0 to disable)")
                  n142 = Less Or Equal?(x=w340, y=w345) -> (x <= y?=w344:bool)
                  n143 = Boolean To (0,1)(Boolean=FALSE) -> (0, 1=w328:i16)
                  n144 = case shown="False" w344 {
                    tunnel: [w349 w353] -> w333
                    tunnel: [w348 0] -> w343
                    tunnel: [0 w351] -> w331
                    tunnel: w330 -> [w349 w353]
                    tunnel: w329 -> [w347 w350]
                    frame True {
                      # "Y"
                      n145 = Negate(x=w347) -> (-x=w348:i32)
                    }
                    frame False {
                      # "X"
                      n146 = Negate(x=w350) -> (-x=w351:i32)
                    }
                  }
                  n147 = call <vilib>:"Digital Write Pin.vi"("Arduino Resource"=w323, "Digital I/O Pin (0)"=u8 13, "Value (0)"=w328, "error in"=w326) -> ("Arduino Resource"=w324:T6, "error out"=w325:errorcluster)  [unwired: 10 in]
                  n148 = call <vilib>:"Stepper Write.vi"("Set Acceleration (0 to disable)"=w332, "Stepper #"=u8 0, "error in"=w325, "Set Speed (Steps per Second)"=w333, "# of Steps to Move"=w343, "Arduino Resource"=w324) -> ("error out"=w339:errorcluster, "Arduino Resource Out"=w338:T6)  [unwired: 4 in]
                  n149 = call <vilib>:"Stepper Write.vi"("Set Acceleration (0 to disable)"=w332, "Stepper #"=u8 1, "error in"=w339, "Set Speed (Steps per Second)"=w333, "# of Steps to Move"=w331, "Arduino Resource"=w338) -> ("error out"=w336:errorcluster, "Arduino Resource Out"=w337:T6)  [unwired: 4 in]
                  n150 = call <vilib>:"Stepper Wait Till Steps Complete.vi"("error in"=w336, "Arduino Resource In"=w337) -> ("error out"=w341:errorcluster, "Arduino Resource Out"=w342:T6)  [unwired: 8 in]
                }
                frame True {
                  n151 = Wait (ms)(milliseconds to wait=u32 1) -> ()  [unwired: 1 out]
                }
              }
            }
            n152 = Bundle By Name(cluster=w291, "Arduino Resource"=w281) -> (w300:T5)
            n153 = Merge Errors(w303, w280) -> (w287:errorcluster)
          }
          frame "picture processing" {
            n154 = Unbundle By Name(w475) -> ("Threshold"=w476:i32, "Konverziós faktor"=w477:i32)
            n155 = Unbundle By Name(w478) -> ("picture in"=w479:path)
            n156 = control-ref of="Fekete-fehér tükrözött kép"() -> (w486:refnum<vi>)
            n157 = control-ref of="Eredeti kép"() -> (w487:refnum<vi>)
            n158 = control-ref of="XY Graph"() -> (w472:refnum<vi>)
            n159 = call "image process.vi"("Picture in"=w487, "reference in"=w486, "XYGraph Refnum"=w472, "error in (no error)"=w484, "Konverziós faktor"=w477, "picture in"=w479, "Szürkeárnyalat"=w476) -> ("new picture 3"=→"Eredeti kép":picture, "scale maximum"=w489:u32, "régi y felbontás"=→"régi y felbontás":i16, "átméretezett kép"=w488:i32[][], "régi x felbontás"=→"régi x felbontás":i16, "új y felbontás / sorok száma"=w467:i32, "új x felbontás / oszlopok száma"=w466:i32, "new picture 2"=→"Fekete-fehér tükrözött kép":picture, "error out"=w485:errorcluster)  [unwired: 4 in]
            "új y felbontás / sorok száma" <- w467
            "új x felbontás / oszlopok száma" <- w466
            n160 = call "generating sequence of intructions.vi"("scale maximum"=w489, "error in (no error)"=w485, "átméretezett kép"=w488, "új x felbontás / oszlopok száma"=w466, "új y felbontás / sorok száma"=w467) -> ("error out"=w469:errorcluster, "y koordináta"=w483:i32[], "lézer vezérlés"=w482:bool[], "x koordináta"=w481:i32[])  [unwired: 3 in]
            n161 = Bundle By Name(cluster=w478, "új x felbontás / oszlopok száma"=w466, "új y felbontás / sorok száma"=w467, "x koordináta"=w481, "lézer vezérlés"=w482, "y koordináta"=w483) -> (w480:T5)
            n162 = Enqueue Element(queue=w468, element=States."idle" ("enum"), error in (no error)=w469) -> (error out=w470:errorcluster)  [unwired: 1 in, 2 out]
          }
          frame "arduino init" {
            n163 = local read "Szimuláció ON/OFF"() -> (w504:bool)
            n164 = case shown="False" w504 {
              tunnel: [w506 w508] -> w501
              tunnel: [w505 errorcluster {"status"=FALSE, "code"=0, "source"=""} ("error out")] -> w497
              frame False {
                n165 = call "init arduino.vi"("VISA Refnum in"="VISA resource") -> ("error out"=w505:errorcluster, "Arduino Resource"=w506:T6)  [unwired: 9 in]
              }
              frame True {
                w508 = T6 {"VISA resource"="", "Board Type"=enum."Uno", "Connection Type"=enum."USB / Serial", "Bytes Per Packet (15)"=0}  # Arduino Resource
              }
            }
            n166 = Bundle By Name(cluster=w500, "Arduino Resource"=w501) -> (w499:T5)
            n167 = Merge Errors(w498, w497) -> (w495:errorcluster)
            n168 = Enqueue Element(queue=w493, element=States."idle" ("enum"), error in (no error)=w495) -> (error out=w494:errorcluster)  [unwired: 1 in, 2 out]
          }
          frame "engraving" {
            n169 = Unbundle By Name(w511) -> ("Arduino Resource"=w520:T6)
            n170 = Unbundle By Name(w512) -> ("Sebesség"=w516:i32, "Lépés"=w517:i32, "X init"=w519:i32, "Y init"=w518:i32)
            n171 = Add(x=w519, y=w518) -> (x+y=w515:i32)
            n172 = for {
              N: w515 -> [w554]
              tunnel: w519 -> [w560]
              tunnel: [w557] -> w513
              tunnel: [w556] -> w514
              tunnel: w510 -> [w559]
              tunnel: w520 -> [w558]
              tunnel: w516 -> [w552]
              tunnel: w517 -> [w551]
              i -> [w555]
              # "X és Y inicializálása a kép kiinduló pontjára"
              n173 = Increment(x=w555) -> (x+1=w553:i32)
              n174 = Not Equal?(x=w554, y=w553) -> (x != y?=w549:bool)
              n175 = local write "Inicializálás a kezdõpontra"(w549) -> ()
              n176 = local read "Szimuláció ON/OFF"() -> (w550:bool)
              n177 = case shown="False" w550 {
                tunnel: w560 -> [w584 _]
                tunnel: w559 -> [w564 w593]
                tunnel: w558 -> [w561 w592]
                tunnel: [w581 w592] -> w557
                tunnel: [w580 w593] -> w556
                tunnel: w553 -> [w579 _]
                tunnel: w552 -> [w569 _]
                tunnel: w551 -> [w568 _]
                frame False {
                  w571 = i16 0 ("Set Acceleration (0 to disable)")
                  n178 = Less Or Equal?(x=w579, y=w584) -> (x <= y?=w583:bool)
                  n179 = Boolean To (0,1)(Boolean=FALSE) -> (0, 1=w567:i16)
                  n180 = case shown="False" w583 {
                    tunnel: [w587 w590] -> w572
                    tunnel: [w585 0] -> w582
                    tunnel: [0 w588] -> w570
                    tunnel: w569 -> [w587 w590]
                    tunnel: w568 -> [w585 w588]
                    frame True {
                      # "Y"
                    }
                    frame False {
                      # "X"
                    }
                  }
                  n181 = call <vilib>:"Digital Write Pin.vi"("Arduino Resource"=w561, "Digital I/O Pin (0)"=u8 13, "Value (0)"=w567, "error in"=w564) -> ("Arduino Resource"=w563:T6, "error out"=w562:errorcluster)  [unwired: 10 in]
                  n182 = call <vilib>:"Stepper Write.vi"("Set Acceleration (0 to disable)"=w571, "Stepper #"=u8 0, "error in"=w562, "Set Speed (Steps per Second)"=w572, "# of Steps to Move"=w582, "Arduino Resource"=w563) -> ("error out"=w578:errorcluster, "Arduino Resource Out"=w577:T6)  [unwired: 4 in]
                  n183 = call <vilib>:"Stepper Write.vi"("Set Acceleration (0 to disable)"=w571, "Stepper #"=u8 1, "error in"=w578, "Set Speed (Steps per Second)"=w572, "# of Steps to Move"=w570, "Arduino Resource"=w577) -> ("error out"=w575:errorcluster, "Arduino Resource Out"=w576:T6)  [unwired: 4 in]
                  n184 = call <vilib>:"Stepper Wait Till Steps Complete.vi"("error in"=w575, "Arduino Resource In"=w576) -> ("error out"=w580:errorcluster, "Arduino Resource Out"=w581:T6)  [unwired: 8 in]
                }
                frame True {
                  n185 = Wait (ms)(milliseconds to wait=u32 1) -> ()  [unwired: 1 out]
                }
              }
            }
            n186 = Unbundle By Name(w512) -> ("Lépés"=w530:i32, "Sebesség"=w529:i32)
            n187 = Unbundle By Name(w511) -> ("x koordináta"=w545:i32[], "lézer vezérlés"=w544:bool[], "y koordináta"=w543:i32[], "új x felbontás / oszlopok száma"=w542:i32)
            n188 = invoke on="XY Graph" class="XYGraph (strict)" method="Reinit To Default"() -> (error out=w531:errorcluster)  [unwired: 3 in, 2 out]
            n189 = To Long Integer(number=w545) -> (32bit integer=w541:i32[])
            n190 = for {
              N -> [w660]
              tunnel: w544 -> [w662] mode=indexing
              tunnel: w543 -> [w648] mode=indexing
              tunnel: w541 -> [w649] mode=indexing
              tunnel: w542 -> [w666]
              shift-right: [w645] -> _
              shift-left: cluster{i32, i32}[] [] -> [w646]
              tunnel: [w649] -> w526
              tunnel: [w648] -> w521
              tunnel: [w663] -> w536
              tunnel: [w650] -> w537
              tunnel: w513 -> [w665]
              tunnel: w514 -> [w651]
              tunnel: w531 -> [_]
              tunnel: w530 -> [w643]
              tunnel: w529 -> [w642]
              i -> [w659]
              stop <- w652 stop-if-true
              # "A megmunkálás vezérlése és pillanatnyi helyzetének visszaigazolása"
              n191 = Increment(x=w659) -> (x+1=w657:i32)
              n192 = Equal?(x=w660, y=w657) -> (x = y?=w658:bool)
              "Megmunkálás kész" <- w658
              n193 = case shown="False" w662 {
                tunnel: w649 -> [_ w715]
                tunnel: [_ w715] -> w670
                tunnel: w648 -> [_ w716]
                tunnel: [_ w716] -> w669
                tunnel: [TRUE FALSE] -> w667
                frame False {
                }
                frame True {
                }
              }
              n194 = local read "Szimuláció ON/OFF"() -> (w661:bool)
              n195 = case shown="False" w661 {
                tunnel: w649 -> [w694 _]
                tunnel: w666 -> [w693 _]
                tunnel: w651 -> [w691 w710]
                tunnel: w665 -> [w690 w711]
                tunnel: [w686 w710] -> w650
                tunnel: [w685 w711] -> w663
                tunnel: w662 -> [w684 _]
                tunnel: w657 -> [w683 _]
                tunnel: w643 -> [w671 _]
                tunnel: w642 -> [w672 _]
                frame False {
                  w677 = i16 0 ("Set Acceleration (0 to disable)")
                  n196 = Boolean To (0,1)(Boolean=w684) -> (0, 1=w692:i16)
                  n197 = Quotient & Remainder(x=w683, y=w693) -> (x-y*floor(x/y)=w696:i32)  [unwired: 1 out]
                  n198 = Equal?(x=w696, y=0) -> (x = y?=w695:bool)
                  n199 = call <vilib>:"Digital Write Pin.vi"("Arduino Resource"=w690, "Digital I/O Pin (0)"=u8 13, "Value (0)"=w692, "error in"=w691) -> ("Arduino Resource"=w689:T6, "error out"=w688:errorcluster)  [unwired: 10 in]
                  n200 = case shown="True" w695 {
                    tunnel: w694 -> [_ w707]
                    tunnel: w693 -> [_ w706]
                    tunnel: [w700 w704] -> w675
                    tunnel: [0 w705] -> w673
                    tunnel: [w699 0 ("Lépés")] -> w674
                    tunnel: w672 -> [w700 w704]
                    tunnel: w671 -> [w699 w702]
                    frame True {
                      # "Y"
                    }
                    frame False {
                      # "X"
                      n201 = Negate(x=w702) -> (-x=w701:i32)
                      n202 = Less?(x=w707, y=w706) -> (x < y?=w708:bool)
                      n203 = Select(t=w702, s=w708, f=w701) -> (s? t:f=w705:i32)
                    }
                  }
                  n204 = call <vilib>:"Stepper Write.vi"("Set Acceleration (0 to disable)"=w677, "Stepper #"=u8 0, "error in"=w688, "Set Speed (Steps per Second)"=w675, "# of Steps to Move"=w674, "Arduino Resource"=w689) -> ("error out"=w679:errorcluster, "Arduino Resource Out"=w680:T6)  [unwired: 4 in]
                  n205 = call <vilib>:"Stepper Write.vi"("Set Acceleration (0 to disable)"=w677, "Stepper #"=u8 1, "error in"=w679, "Set Speed (Steps per Second)"=w675, "# of Steps to Move"=w673, "Arduino Resource"=w680) -> ("error out"=w681:errorcluster, "Arduino Resource Out"=w682:T6)  [unwired: 4 in]
                  n206 = call <vilib>:"Stepper Wait Till Steps Complete.vi"("error in"=w681, "Arduino Resource In"=w682) -> ("error out"=w686:errorcluster, "Arduino Resource Out"=w685:T6)  [unwired: 8 in]
                }
                frame True {
                  n207 = Wait (ms)(milliseconds to wait=u32 1) -> ()  [unwired: 1 out]
                }
              }
              n208 = Bundle(w649, w648) -> (w641:cluster{i32, i32})  [unwired: 1 in]
              n209 = Bundle(w670, w669) -> (w647:cluster{i32, i32})  [unwired: 1 in]
              n210 = Not(x=w658) -> (.not. x?=w655:bool)
              n211 = And(x=w667, y="Megmunkálás leállítása") -> (x .and. y?=w653:bool)
              n212 = Exclusive Or(1:"Megmunkálás leállítása", 2:w655) -> (0:→"Megmunkálás folyamatban":bool)
              n213 = Or(x=w653, y=w650) -> (x .or. y?=w652:bool)
              n214 = And(x="Felfüggesztés/Folytatás", y=w667) -> (x .and. y?=w668:bool)
              n215 = case shown="False" w668 {
                frame False {
                  # "Continue consumer loop"
                }
                frame True {
                  # "Pause consumer loop"
                  n216 = while {
                    stop <- w712 continue-if-true
                    n217 = local read "Felfüggesztés/Folytatás"() -> (w712:bool)
                  }
                }
              }
              n218 = Build Array (concatenate)(w646, w647) -> (w645:cluster{i32, i32}[])
              n219 = Build Array (concatenate)(w645, w641) -> (→"XY Graph":cluster{i32, i32}[])
            }
            n220 = Enqueue Element(queue=w547, element=States."report" ("enum"), error in (no error)=w510) -> (error out=w539:errorcluster)  [unwired: 1 in, 2 out]
            n221 = Unbundle By Name(w512) -> ("Sebesség"=w528:i32, "Lépés"=w527:i32, "X init"=w525:i32, "Y init"=w523:i32)
            n222 = Add(x=w525, y=w526) -> (x+y=w524:i32)
            n223 = Add(x=w521, y=w523) -> (x+y=w522:i32)
            n224 = Add(x=w524, y=w522) -> (x+y=w535:i32)
            n225 = for {
              N: w535 -> [w598]
              tunnel: w524 -> [w605]
              tunnel: [w602] -> w533
              tunnel: [w601] -> w534
              tunnel: w537 -> [w604]
              tunnel: w536 -> [w603]
              tunnel: w528 -> [w595]
              tunnel: w527 -> [w594]
              i -> [w599]
              # "X és Y inicializálása a globális kiindulópontra\na megmunkálás végeztével"
              n226 = Increment(x=w599) -> (x+1=w597:i32)
              n227 = Not Equal?(x=w598, y=w597) -> (x != y?=→"Inicializálás a kezdõpontra":bool)
              n228 = local read "Szimuláció ON/OFF"() -> (w600:bool)
              n229 = case shown="False" w600 {
                tunnel: w605 -> [w629 _]
                tunnel: w604 -> [w610 w640]
                tunnel: w603 -> [w607 w639]
                tunnel: [w626 w639] -> w602
                tunnel: [w625 w640] -> w601
                tunnel: w597 -> [w624 _]
                tunnel: w595 -> [w614 _]
                tunnel: w594 -> [w613 _]
                frame False {
                  w616 = i16 0 ("Set Acceleration (0 to disable)")
                  n230 = Less Or Equal?(x=w624, y=w629) -> (x <= y?=w628:bool)
                  n231 = Boolean To (0,1)(Boolean=FALSE) -> (0, 1=w612:i16)
                  n232 = case shown="False" w628 {
                    tunnel: [w633 w637] -> w617
                    tunnel: [w632 0] -> w627
                    tunnel: [0 w635] -> w615
                    tunnel: w614 -> [w633 w637]
                    tunnel: w613 -> [w631 w634]
                    frame True {
                      # "Y"
                      n233 = Negate(x=w631) -> (-x=w632:i32)
                    }
                    frame False {
                      # "X"
                      n234 = Negate(x=w634) -> (-x=w635:i32)
                    }
                  }
                  n235 = call <vilib>:"Digital Write Pin.vi"("Arduino Resource"=w607, "Digital I/O Pin (0)"=u8 13, "Value (0)"=w612, "error in"=w610) -> ("Arduino Resource"=w608:T6, "error out"=w609:errorcluster)  [unwired: 10 in]
                  n236 = call <vilib>:"Stepper Write.vi"("Set Acceleration (0 to disable)"=w616, "Stepper #"=u8 0, "error in"=w609, "Set Speed (Steps per Second)"=w617, "# of Steps to Move"=w627, "Arduino Resource"=w608) -> ("error out"=w623:errorcluster, "Arduino Resource Out"=w622:T6)  [unwired: 4 in]
                  n237 = call <vilib>:"Stepper Write.vi"("Set Acceleration (0 to disable)"=w616, "Stepper #"=u8 1, "error in"=w623, "Set Speed (Steps per Second)"=w617, "# of Steps to Move"=w615, "Arduino Resource"=w622) -> ("error out"=w620:errorcluster, "Arduino Resource Out"=w621:T6)  [unwired: 4 in]
                  n238 = call <vilib>:"Stepper Wait Till Steps Complete.vi"("error in"=w620, "Arduino Resource In"=w621) -> ("error out"=w625:errorcluster, "Arduino Resource Out"=w626:T6)  [unwired: 8 in]
                }
                frame True {
                  n239 = Wait (ms)(milliseconds to wait=u32 1) -> ()  [unwired: 1 out]
                }
              }
            }
            n240 = Merge Errors(w539, w534) -> (w540:errorcluster)
            n241 = Bundle By Name(cluster=w511, "Arduino Resource"=w533) -> (w538:T5)
          }
          frame "report" {
            n242 = Unbundle By Name(w732) -> ("config"=w719:path, "report"=w720:path)
            n243 = Unbundle By Name(w725) -> ("Megjegyzések"=w724:string)
            n244 = Get Date/Time In Seconds() -> (seconds since 1Jan1904=w726:timestamp)
            n245 = Format Date/Time String(seconds (now)=w726) -> (date/time string=w729:string)  [unwired: 2 in]
            n246 = Strip Path(path=w719) -> (name=w730:string)  [unwired: 1 out]
            n247 = Build Array(w729, w730, w724) -> (w728:string[])
            n248 = call-poly <vilib>:"Write Delimited Spreadsheet.vi"("file path (dialog if empty)"=w720, "format (%s)"="%s", "1D data"=w728, "append to file? (new file:F)"=TRUE, "error in (no error)"=w722, "transpose? (no:F)"=FALSE ("append to file? (new file:F)"), "delimiter (\\t)"="\t") -> ("error out"=w723:errorcluster)  [unwired: 7 in, 1 out]
            n249 = Enqueue Element(queue=w733, element=States."idle" ("enum"), error in (no error)=w723) -> (error out=w734:errorcluster)  [unwired: 1 in, 2 out]
          }
          frame "load control panel" {
            n250 = call <vilib>:"Application Directory.vi"() -> ("Application Directory"=w744:path)
            n251 = call "Kezelõpult betöltése"("start path"=w744, "button label"="Kezelõpult betöltése", "error in"=w742) -> ("selected path"=w736:path, "error out"=w739:errorcluster)  [unwired: 9 in, 2 out]
            n252 = Unbundle By Name(w738) -> ("config"=w737:path)
            n253 = case shown="No Error" w739 {
              selector: w739 -> [w752 w767]
              tunnel: w747 -> [w758 _]
              tunnel: [w757 w765] -> w746
              tunnel: [w753 w766] -> w740
              tunnel: w737 -> [_ w766]
              tunnel: w736 -> [w751 _]
              frame No Error {
                n254 = Open/Create/Replace File(file path (use dialog)=w751, error in=w752, operation (0:open)=T8."open") -> (refnum out=w761:refnum<file>, error out=w762:errorcluster)  [unwired: 3 in, 1 out]
                n255 = Read from Text File(file (use dialog)=w761, error in=w762) -> (refnum out=w759:refnum<file>, text=w763:string, error out=w764:errorcluster)  [unwired: 2 in, 1 out]
                n256 = Unflatten From XML(xml string=w763, type=w758, error in (no error)=w764) -> (value=w754:T2, error out=w755:errorcluster)
                n257 = property on="Kezelõpult" class="Clust (strict)"(error in=w755, "Value"=w754) -> (error out=w756:errorcluster)  [unwired: 1 in, 1 out]
                n258 = Close File(refnum=w759, error in=w756) -> (path=w753:path, error out=w757:errorcluster)
              }
              frame Error {
                n259 = call <vilib>:"Clear Errors.vi"("error in (no error)"=w767, "specific error code to clear (0: all)"=43) -> ("error out"=w765:errorcluster)  [unwired: 4 in, 1 out]
              }
            }
            n260 = Bundle By Name(cluster=w738, "config"=w740) -> (w741:T5)
            n261 = Enqueue Element(queue=w749, element=States."idle" ("enum"), error in (no error)=w746) -> (error out=w750:errorcluster)  [unwired: 1 in, 2 out]
          }
          frame "save control panel" {
            n262 = call <vilib>:"Application Directory.vi"() -> ("Application Directory"=w776:path)
            n263 = call "Kezelõpult mentése"("start path"=w776, "button label"="Kezelõpult mentése", "error in"=w775) -> ("selected path"=w774:path, "error out"=w771:errorcluster)  [unwired: 9 in, 2 out]
            n264 = Unbundle By Name(w770) -> ("config"=w769:path)
            n265 = case shown="No Error" w771 {
              selector: w771 -> [w784 w797]
              tunnel: [w788 w796] -> w781
              tunnel: w780 -> [w787 _]
              tunnel: w774 -> [w786 _]
              tunnel: [w785 w795] -> w773
              tunnel: w769 -> [_ w795]
              frame No Error {
                n266 = Open/Create/Replace File(file path (use dialog)=w786, error in=w784, operation (0:open)=T8."open") -> (refnum out=w794:refnum<file>, error out=w793:errorcluster)  [unwired: 3 in, 1 out]
                n267 = Flatten To XML(anything=w787) -> (xml string=w789:string)
                n268 = Write to Text File(file (use dialog)=w794, text=w789, error in=w793) -> (refnum out=w791:refnum<file>, error out=w790:errorcluster)  [unwired: 1 in, 1 out]
                n269 = Close File(refnum=w791, error in=w790) -> (path=w785:path, error out=w788:errorcluster)
              }
              frame Error {
                n270 = call <vilib>:"Clear Errors.vi"("error in (no error)"=w797, "specific error code to clear (0: all)"=43) -> ("error out"=w796:errorcluster)  [unwired: 4 in, 1 out]
              }
            }
            n271 = Bundle By Name(cluster=w770, "config"=w773) -> (w772:T5)
            n272 = Enqueue Element(queue=w779, element=States."idle" ("enum"), error in (no error)=w781) -> (error out=w783:errorcluster)  [unwired: 1 in, 2 out]
          }
          frame "idle", Default {
          }
          frame "stop" {
            n273 = local read "Szimuláció ON/OFF"() -> (w803:bool)
            n274 = Unbundle By Name(w807) -> ("Arduino Resource"=w805:T6)
            n275 = case shown="False" w803 {
              tunnel: [w811 w814] -> w806
              tunnel: w805 -> [w813 _]
              tunnel: w804 -> [w812 w814]
              frame False {
                n276 = call "close arduino.vi"("error in (no error)"=w812, "Arduino Resource Out"=w813) -> ("error out"=w811:errorcluster)  [unwired: 9 in]
              }
              frame True {
              }
            }
          }
        }
      }
      frame Error {
        n277 = local read "Szimuláció ON/OFF"() -> (w815:bool)
        n278 = Unbundle By Name(w817) -> ("Arduino Resource"=w816:T6)
        n279 = case shown="False" w815 {
          tunnel: [w825 w828] -> w819
          tunnel: w818 -> [w827 w828]
          tunnel: w816 -> [w826 _]
          frame False {
            n280 = call "close arduino.vi"("error in (no error)"=w827, "Arduino Resource Out"=w826) -> ("error out"=w825:errorcluster)  [unwired: 9 in]
          }
          frame True {
          }
        }
        n281 = Generate User Event(user event=w824, event data cluster=w818) -> (user event out=w823:refnum<user-event>)  [unwired: 2 in, 1 out]
        n282 = Merge Errors(w818, w819) -> (w820:errorcluster)
      }
    }
  }
  n283 = Merge Errors(w25, w15) -> (w18:errorcluster)
  n284 = Release Queue(queue=w17, error in (no error)=w18) -> (error out=w24:errorcluster)  [unwired: 1 in, 2 out]
  n285 = Unregister For Events(event registration refnum=w19, error in=w24) -> (error out=w23:errorcluster)
  n286 = Destroy User Event(user event=w9, error in=w23) -> (error out=w10:errorcluster)
  n287 = call <vilib>:"Simple Error Handler.vi"("error in (no error)"=w10) -> ()  [unwired: 4 in, 5 out]
